vi "GFITS_Main.vi"() -> ()   [LabVIEW 2016]
doc: "Main VI for the TCS P60 interface"
uses:
  Common/public/vis/CMN_FVAR_action.ctl
  DBSHAND/private/vis/DatabaseHand_Element_Set(string).vi
  private/vis/GFITS_Gbls.vi
  DBSHAND/private/vis/DatabaseHand_Element_Get(string).vi
  DBSHAND/private/vis/DatabaseHand_Element_Get(bool).vi
  DBSHAND/private/vis/DatabaseHand_Element_Get(I32).vi
  DBSHAND/private/vis/DatabaseHand_Element_Set(I32).vi
  DBSHAND/private/vis/DatabaseHand_Element_Set(bool).vi
  DBSHAND/private/vis/DatabaseHand_Element_Get(path).vi
panel:
  in  "ignorename":string
  in  "testbname":string="test"
  in  "testdir":path=path "/tmp"
  out "tmpname":bool
  in  "postimg":string="none"
  in  "lognetfile":path
  in  "lognet":bool
  in  "defexts":bool=TRUE
  in  "imlog":bool
  in  "maxlistsize":i32=200
  in  "geomhdrmode":string="dynamic"
  in  "hdrmode":string="dynamic"
  in  "hdrprealloc":string="auto"
  in  "imnumformat":string="%04d"
  in  "waitstats":u32
  in  "preimg":string="none"
  in  "logfilepp":path
  in  "logpp":bool
  in  "postproc":string
  out "multiple extensions":bool
  out "after expid":string
  in  "filemsg":string
  in  "headers":bool=TRUE
  out "expID":string
  in  "asyncs":bool
  in  "imlogpath":path
  in  "cmdport2":u16=4062
  out "mImpath":string
  in  "nodeID":string
  in  "netenable":bool
  in  "cmdport":u16
  in  "saveconfig":bool
  out "image name out":string
  out "imretries":i32=20
  in  "log":bool
  in  "logfile":path
  in  "def_head_tim":string="after"
  out "amplifiers":u64
  in  "commands2exec":string
  in  "hdrfile":path
  out "ReadMode":string
  out "number of keywords":i32[](array[numeric])
  out "file reference":u64
  out "image size":u32
  in  "image data":T1
  in  "cmd struct":T2
  out "error out":errorcluster
  in  "Initialization Variables":string[][](table)=[["HDRFILE", "path", "GFITS_Main.vi", "hdrfile", "", "PATH"], ["HDRFILE", "prealloc", "GFITS_Main.vi", "hdrprealloc", "", "STR"], ["HDRFILE", "geommode", "GFITS_Main.vi", "geomhdrmode", "", "STR"], ["HDRFILE", "defmultext", "GFITS_Main.vi", "defexts", "", "BOOL"], ["HDRFILE", "mode", "GFITS_Main.vi", "hdrmode", "", "STR"], ["MISC", "commands", "GFITS_Main.vi", "commands2exec", "none", "STR"], ["MISC", "headtiming", "GFITS_Main.vi", "def_head_tim", "after", "STR"], ["MISC", "autosavecfg", "GFITS_Main.vi", "saveconfig", "", "BOOL"], ["MISC", "asyncmsg", "GFITS_Main.vi", "asyncs", "", "BOOL"], ["MISC", "filemsg", "GFITS_Main.vi", "filemsg", "", "STR"], ["MISC", "imnumformat", "GFITS_Main.vi", "imnumformat", "", "STR"], ["MISC", "testdir", "GFITS_Main.vi", "testdir", "", "PATH"], ["MISC", "testbname", "GFITS_Main.vi", "testbname", "", "STR"], ["MISC", "ignorename", "GFITS_Main.vi", "ignorename", "", "STR"], ["LOG", "file", "GFITS_Main.vi", "logfile", "none", "PATH"], ["LOG", "log", "GFITS_Main.vi", "log", "FALSE", "BOOL"], ["LOG", "imlogfile", "GFITS_Main.vi", "imlogpath", "", "PATH"], ["LOG", "imlog", "GFITS_Main.vi", "imlog", "", "BOOL"], ["LOG", "maxlistsize(kb)", "GFITS_Main.vi", "maxlistsize", "", "I32"], ["NetComms", "port", "GFITS_Main.vi", "cmdport", "", "U16"], ["NetComms", "port2", "GFITS_Main.vi", "cmdport2", "", "U16"], ["NetComms", "enable", "GFITS_Main.vi", "netenable", "", "BOOL"], ["NetComms", "log", "GFITS_Main.vi", "lognet", "", "BOOL"], ["NetComms", "logfile", "GFITS_Main.vi", "lognetfile", "", "PATH"], ["PostProc", "cmd", "GFITS_Main.vi", "postproc", "", "STR"], ["PostProc", "log", "GFITS_Main.vi", "logpp", "", "BOOL"], ["PostProc", "file", "GFITS_Main.vi", "logfilepp", "", "PATH"], ["PostImg", "cmd", "GFITS_Main.vi", "postimg", "", "STR"], ["PreImg", "cmd", "GFITS_Main.vi", "preimg", "", "STR"]]
  in  "error in":errorcluster
  out "ConfigFile":path=path "/home/ArcVIEW/Modules/TCSP60/config/TCSP60_Default.cfg"
  in  "ModuleName":string="GFITS"
  out "Command":string
  out "stopped":bool=TRUE
  out "Reply to":string
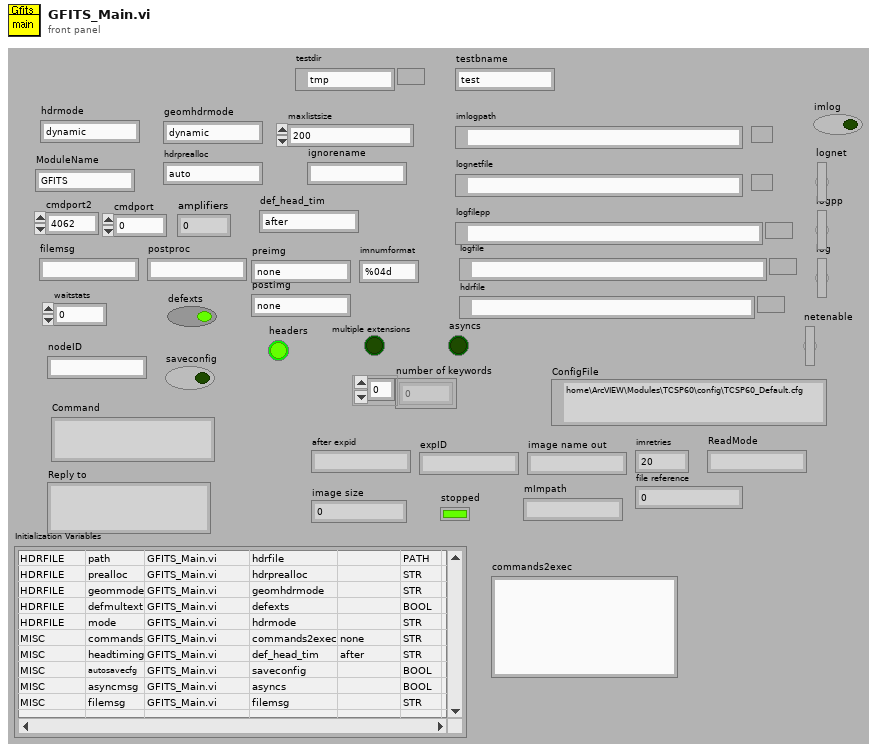
[diagram p1: front panel]
types:
  T1 = cluster{"location":u64, "eleRead":u32[], "data":u16[]}
  T2 = cluster{"command":string, "data":string, "responseQ":string, "nodeID":string}
  T3 = cluster{"name":string, "Path":path, "bitpix":i8, "naxis":u8, "naxes":u32[], "datatype":u16, "multiple extensions":bool, "hdutype":u16, "writeToDisk":bool, "num_of_ext":u8, "file ref":i32, "createnewimage":bool}
  T4 = typedef "CMN_FVAR_action.ctl" = enum16{"read", "write"}
  T5 = typedef "DatabaseHand_RefNum.ctl" = refnum<vi>
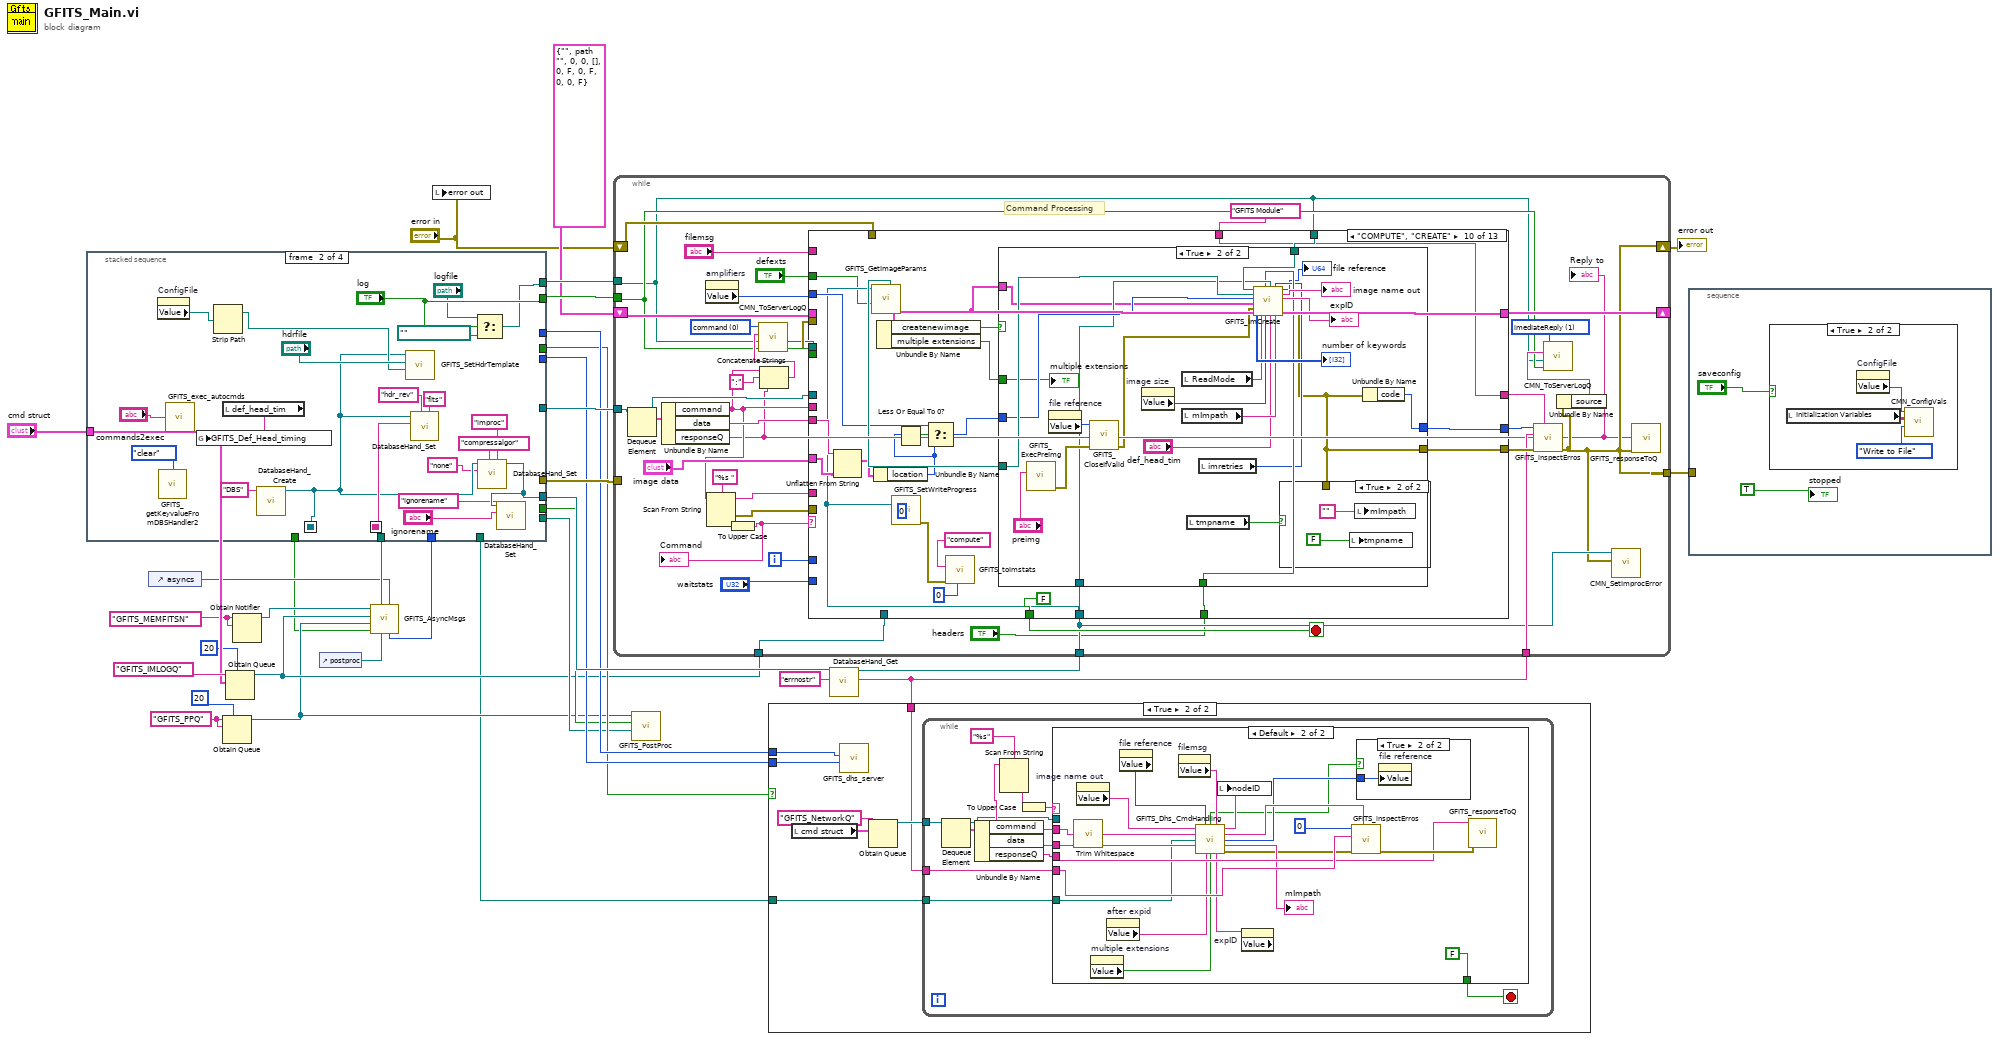
[diagram p0: block diagram]
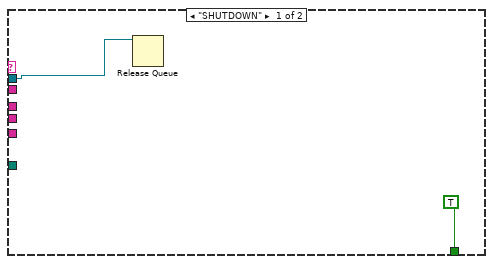
[diagram p3: hidden frame]
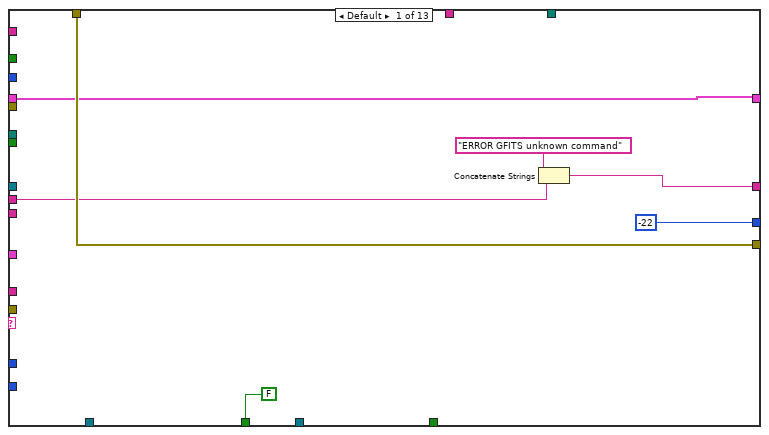
[diagram p6: hidden frame]
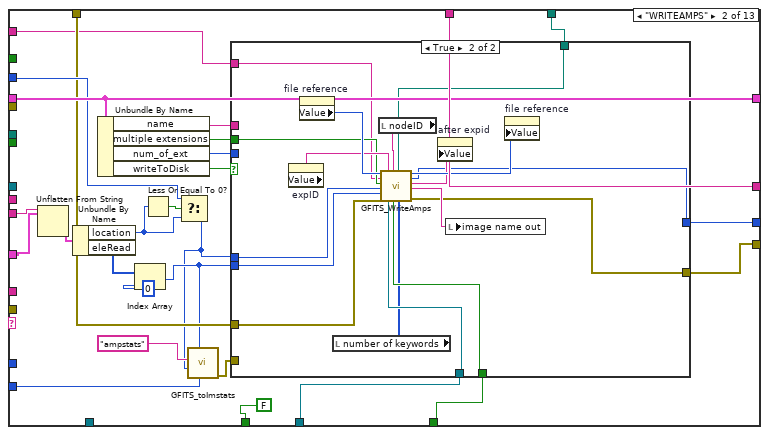
[diagram p7: hidden frame]
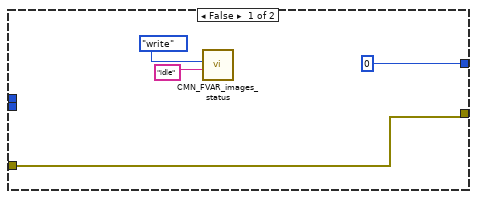
[diagram p8: hidden frame]
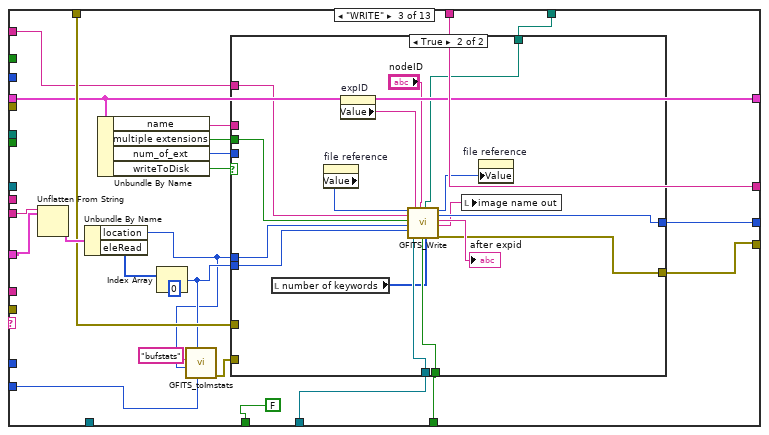
[diagram p9: hidden frame]
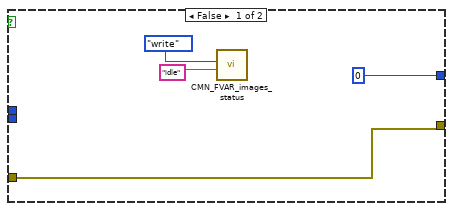
[diagram p10: hidden frame]
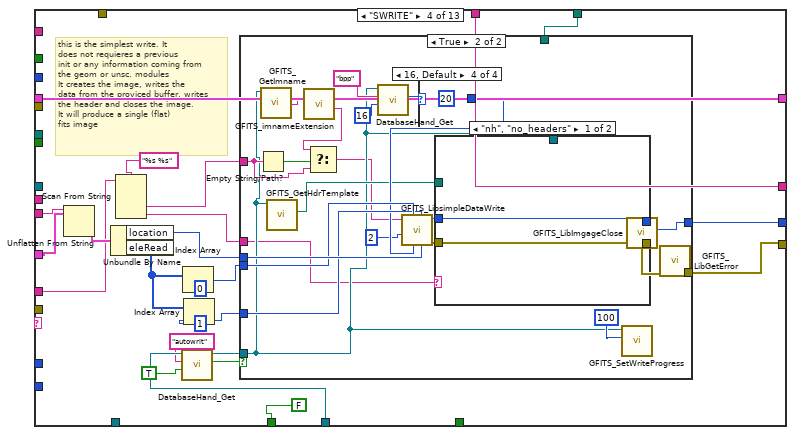
[diagram p11: hidden frame]
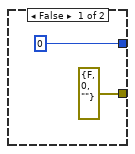
[diagram p12: hidden frame]
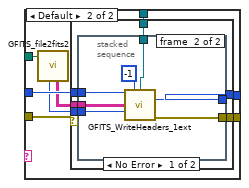
[diagram p13: hidden frame]
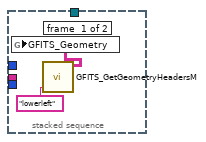
[diagram p14: hidden frame]
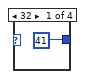
[diagram p16: hidden frame]
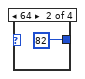
[diagram p17: hidden frame]
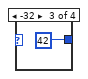
[diagram p18: hidden frame]
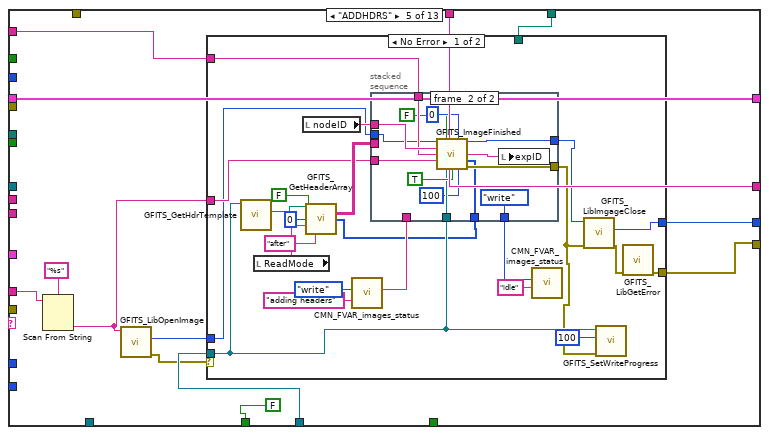
[diagram p19: hidden frame]
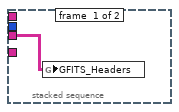
[diagram p20: hidden frame]
diagram:
  w14 = "GFITS_PPQ" ("name (unnamed)")
  w16 = "GFITS_MEMFITSN" ("name (unnamed)")
  n1 = stacked-sequence {
    seq-local: [w39 _ _ _] -> [_ w57 _ _]
    seq-local: [_ w50 _ _] -> [_ _ w69 _]
    tunnel: [w36 _ _ _] -> w32
    tunnel: [_ w48 _ _] -> w31
    tunnel: [_ "log" _ _] -> w30
    tunnel: [_ w60 _ _] -> w29
    tunnel: [w37 _ _ _] -> w28
    tunnel: [_ _ "cmdport" _] -> w21
    tunnel: [_ _ "netenable" _] -> w20
    tunnel: [_ _ "cmdport2" _] -> w22
    tunnel: [_ _ "imlogpath" _] -> w8
    tunnel: "cmd struct" -> [w35 _ _ _]
    tunnel: [_ _ "logpp" _] -> w13
    tunnel: [_ _ "logfilepp" _] -> w12
    tunnel: [_ _ w79 _] -> w3
    tunnel: [_ _ "imlog" _] -> w2
    tunnel: [_ _ _ "lognetfile"] -> w1
    frame #0 {
      # "Initialization"
      n2 = call "CMN_FVAR_images_status.vi"("value in"="idle", "action"=CMN_FVAR_action."write") -> ()  [unwired: 9 out]
      n3 = Current VI's Path() -> (path=w41:path)
      n4 = call "CMN_testpath.vi"("ModuleName"="ModuleName", "caller Path"=w41) -> ("ConfigFile"=w43:path)  [unwired: 1 in, 8 out]
      "ConfigFile" <- w43
      n5 = local write "stopped"(FALSE ("stopped")) -> ()
      n6 = call "CMN_modinfo.vi"("full"=FALSE, "caller path"=w41) -> ("INFO"=w39:string)  [unwired: 1 in, 8 out]
      n7 = Obtain Queue(name (unnamed)="GFITS_INTERNALQ", element data type=w35) -> (queue out=w37:refnum<queue>, error out=w36:errorcluster)  [unwired: 3 in, 1 out]
      n8 = call "CMN_ConfigVals.vi"("ConfigVariables"="Initialization Variables", "configuration file path"=w43) -> ()  [unwired: 2 in, 8 out]
    }
    frame #1 {
      n9 = property on="ConfigFile" class="Path"() -> ("Value"=w54:path)  [unwired: 2 in, 2 out]
      n10 = call "GFITS_getKeyvalueFromDBSHandler2.vi"("action"=enum16{"get", "clear"}."clear") -> ()  [unwired: 8 in, 7 out]
      n11 = call "GFITS_exec_autocmds.vi"("commands2exec"="commands2exec") -> ()
      n12 = Strip Path(path=w54) -> (stripped path=w53:path)  [unwired: 1 out]
      n13 = local read "def_head_tim"() -> (w56:string)
      n14 = global write "GFITS_Gbls.vi" "GFITS_Def_Head_timing"(w56) -> ()
      n15 = call "DatabaseHand_Create.vi"("Name"="DBS") -> ("Database RefNum out"=w50:T5)  [unwired: 1 in, 9 out]
      n16 = call "GFITS_SetHdrTemplate.vi"("ref path"=w53, "path"="hdrfile", "Database RefNum"=w50) -> ()  [unwired: 9 out]
      n17 = call-poly "DatabaseHand_Set.vi"("group"="fits", "name"="hdr_rev", "value"=w57, "Database RefNum in"=w50) -> ()  [unwired: 4 in, 4 out]
      n18 = Select(t="logfile", s="log", f=path "") -> (s? t:f=w60:path)
      n19 = call-poly "DatabaseHand_Set.vi"("group"="improc", "name"="compressalgor", "value"="none", "Database RefNum in"=w50) -> ("Database RefNum out"=w48:T5)  [unwired: 4 in, 3 out]
      n20 = call-poly "DatabaseHand_Set.vi"("name"="ignorename", "value"="ignorename", "Database RefNum in"=w48) -> ()  [unwired: 5 in, 4 out]
    }
    frame #2 {
      n21 = property on="preimg" class="Str"() -> ("Value"=w73:string)  [unwired: 2 in, 2 out]
      n22 = call "GFITS_ParsePostProc.vi"("postproc in"=w73) -> ("postproc out"=w72:string)  [unwired: 10 out]
      n23 = call "GFITS_ParsePostProc.vi"("postproc in"="postproc") -> ("postproc out"=w75:string)  [unwired: 10 out]
      n24 = call "GFITS_ParsePostProc.vi"("postproc in"="postimg") -> ("postproc out"=w71:string)  [unwired: 10 out]
      n25 = case shown="False" "lognet" {
        frame False {
          n26 = property on="lognetfile" class="Path"("Value"=path "") -> ()  [unwired: 2 in, 2 out]
        }
        frame True {
        }
      }
      n27 = property on="postproc" class="Str"("Value"=w75) -> ()  [unwired: 2 in, 2 out]
      n28 = property on="preimg" class="Str"("Value"=w72) -> ()  [unwired: 2 in, 2 out]
      n29 = call "GFITS_VAR_postImgScript.vi"("script name in"=w71, "action"=enum16{"read", "write"}."write") -> ()  [unwired: 14 out]
      n30 = call "GFITS_SetImNumFormat.vi"("imnumformat"="imnumformat", "Database RefNum out"=w69) -> ()  [unwired: 1 in, 9 out]
      n31 = call "GFITS_LibInitExtensions.vi"() -> ()  [unwired: 1 in, 11 out]
      n32 = Multiply(x="maxlistsize", y=1024) -> (x*y=w79:i32)
      n33 = call "GFITS_SetTestVars.vi"("testbname"="testbname", "testdir"="testdir", "Database RefNum in"=w69) -> ()  [unwired: 9 out]
    }
    frame #3 {
      n34 = call <vilib>:"Trim Whitespace.vi"("string"="geomhdrmode") -> ("trimmed string"=w92:string)  [unwired: 1 in]
      n35 = call <vilib>:"Trim Whitespace.vi"("string"="hdrmode") -> ("trimmed string"=w99:string)  [unwired: 1 in]
      n36 = call <vilib>:"Trim Whitespace.vi"("string"="hdrprealloc") -> ("trimmed string"=w101:string)  [unwired: 1 in]
      n37 = To Lower Case(string=w92) -> (all lower case string=w91:string)
      n38 = To Lower Case(string=w99) -> (all lower case string=w100:string)
      n39 = To Lower Case(string=w101) -> (all lower case string=w105:string)
      n40 = case shown="\"\", \"auto\", \"dynamic\", Default" w91 {
        tunnel: w92 -> [_ _]
        tunnel: [TRUE ("nkeys in") FALSE ("nkeys in")] -> w95
        frame "static" {
        }
        frame "", "auto", "dynamic", Default {
        }
      }
      n41 = case shown="\"\", \"auto\", \"dynamic\"" w105 {
        tunnel: [w111 -1 ("nkeys in")] -> w103
        tunnel: w101 -> [w114 _]
        frame Default {
          n42 = Scan From String(format string="%d", input string=w114) -> (error out=w113:errorcluster, output 1=w112:i32)  [unwired: 2 in, 3 out]
          n43 = Select(t=-1, s=w113, f=w112) -> (s? t:f=w111:i32)
        }
        frame "", "auto", "dynamic" {
        }
      }
      n44 = case shown="\"\", \"auto\", \"dynamic\", Default" w100 {
        tunnel: w99 -> [_ _]
        tunnel: [TRUE ("nkeys in") FALSE ("nkeys in")] -> w96
        frame "static" {
        }
        frame "", "auto", "dynamic", Default {
        }
      }
      n45 = call "GFITS_VAR_fstaticGeomHdrs.vi"("static in"=w95, "action"=enum16{"read", "write"}."write") -> ()  [unwired: 14 out]
      n46 = call "GFITS_VAR_staticHdrs.vi"("static in"=w96, "action"=enum16{"read", "write"}."write") -> ()  [unwired: 14 out]
      n47 = call "GFITS_VAR_preallocHdrs.vi"("nkeys in"=w103, "action"=enum16{"read", "write"}."write") -> ()  [unwired: 14 out]
    }
  }
  n48 = control-ref of="asyncs"() -> (w7:refnum<vi>)
  n49 = Obtain Queue(max queue size (-1, unlimited)=20, name (unnamed)=w14, element data type=w14) -> (queue out=w9:refnum<queue>)  [unwired: 2 in, 2 out]
  n50 = Obtain Queue(max queue size (-1, unlimited)=20, name (unnamed)="GFITS_IMLOGQ", element data type="cmd struct") -> (queue out=w10:refnum<queue>)  [unwired: 2 in, 2 out]
  n51 = Obtain Notifier(name (unnamed)=w16, notification data type=w16) -> (notifier out=w11:refnum<notifier>)  [unwired: 2 in, 2 out]
  n52 = control-ref of="postproc"() -> (w6:refnum<vi>)
  n53 = call "GFITS_AsyncMsgs.vi"("max imlist size"=w3, "asyncs"=w7, "postproc"=w6, "imlogs"=w8, "imlog"=w2, "PPQ"=w9, "imlogq"=w10, "notifier in"=w11) -> ()  [unwired: 4 out]
  n54 = local write "error out"("error in") -> ()
  n55 = call "GFITS_PostProc.vi"("logpath"=w12, "log"=w13, "queue in"=w9) -> ()  [unwired: 9 out]
  n56 = call-poly "DatabaseHand_Get.vi"("name"="errnostr", "Database RefNum in"=w31) -> ("value"=w19:string, "Database RefNum out"=w24:T5)  [unwired: 3 in, 5 out]
  n57 = while {
    tunnel: w32 -> [_]
    shift-right: [w124] -> w26
    shift-left: "error in" -> [w147]
    shift-right: [w139] -> _
    shift-left: T3 {"name"="", "Path"=path "", "bitpix"=0, "naxis"=0, "naxes"=[], "datatype"=0, "multiple extensions"=FALSE, "hdutype"=0, "writeToDisk"=FALSE, "num_of_ext"=0, "file ref"=0, "createnewimage"=FALSE} ("imageStruct") -> [w141]
    tunnel: [w124] -> w25
    tunnel: w24 -> [w136]
    tunnel: w19 -> [w137]
    tunnel: w29 -> [w128]
    tunnel: w30 -> [w130]
    tunnel: w28 -> [w127]
    tunnel: w10 -> [w121]
    i -> [w153]
    stop <- w154 stop-if-true
    w134 = u16 1 items=["command", "imediateReply", "Callback Reply", "Information"] ("type")
    w135 = u16 0 items=["command", "imediateReply", "Callback Reply", "Information"] ("type")
    # "Command Processing"
    n58 = Dequeue Element(queue=w127) -> (queue out=w125:refnum<queue>, element=w126:T2)  [unwired: 1 in, 3 out]
    n59 = Unbundle By Name(w126) -> ("command"=w123:string, "data"=w145:string, "responseQ"=w122:string)
    "Reply to" <- w122
    n60 = property on="amplifiers" class="DigNum (strict)"() -> ("Value"=w138:u64)  [unwired: 2 in, 2 out]
    n61 = Scan From String(format string="%s ", input string=w123) -> (remaining string=w149:string, error out=w151:errorcluster, output 1=w150:string)  [unwired: 2 in, 2 out]
    n62 = To Upper Case(1:w150) -> (0:w148:string)
    "Command" <- w148
    n63 = Concatenate Strings(w123, ":" ("string"), w122) -> (w132:string)
    n64 = call "CMN_ToServerLogQ.vi"("Log"=w130, "file"=w128, "string"=w132, "type"=w135) -> ("error out"=w129:errorcluster)  [unwired: 2 in, 4 out]
    n65 = case shown="\"COMPUTE\", \"CREATE\"" w148 {
      selector: w148 -> [_ _ _ _ _ _ w423 _ _ _ _ _ _]
      tunnel: [FALSE FALSE FALSE FALSE FALSE FALSE TRUE FALSE FALSE FALSE FALSE FALSE FALSE] -> w154
      tunnel: w151 -> [_ _ _ _ _ _ _ _ _ _ _ _ _]
      tunnel: w153 -> [_ _ _ _ _ _ _ _ _ _ _ _ _]
      tunnel: w149 -> [_ _ _ w257 w339 _ _ _ w453 _ _ _ w1126]
      tunnel: w147 -> [w159 w170 w227 _ _ _ w434 w447 w463 _ _ _ w1124]
      tunnel: [w159 w180 w224 w270 w344 w398 w433 w447 w464 w1049 errorcluster {"status"=FALSE, "code"=0, "source"=""} ("error out") errorcluster {"status"=FALSE, "code"=0, "source"=""} ("error out") w1122] -> w146
      tunnel: w145 -> [_ w188 w233 w277 _ w419 _ _ w455 w1045 _ _ _]
      tunnel: [-22 w182 w226 w272 w346 w416 w432 0 w451 w1048 0 ("return value") 0 ("return value") w1123] -> w144
      tunnel: w123 -> [w157 _ _ _ _ _ _ _ _ _ _ _ _]
      tunnel: "GFITS Module" ("message") -> [_ w181 w225 w271 w345 w420 w436 w442 _ w1029 _ _ _]
      tunnel: [w156 w181 w225 w271 w345 w420 w436 w440 w457 w1029 "aborting write" ("message") "done" ("message") w1121] -> w142
      tunnel: [w155 w179 w223 w269 w343 w403 w435 w439 w465 w1030 w1098 w1109 w1120] -> w139
      tunnel: w141 -> [w155 w179 w223 w269 w343 _ w435 w439 w466 _ w1098 w1109 w1120]
      tunnel: "image data" -> [_ w186 w231 w275 _ w418 _ _ _ w1046 _ _ _]
      tunnel: w138 -> [_ w173 _ _ _ _ _ _ _ w1041 _ _ _]
      tunnel: w136 -> [_ w172 w218 w262 w341 w404 w431 _ w462 w1038 _ w1104 _]
      tunnel: w128 -> [_ _ _ _ _ _ _ _ w460 _ _ _ _]
      tunnel: w130 -> [_ _ _ _ _ _ _ _ w459 _ _ _ _]
      tunnel: w129 -> [_ _ _ _ _ _ _ _ w458 _ _ _ _]
      tunnel: w128 -> [_ w171 w217 w268 w342 _ _ _ _ w1037 _ _ _]
      tunnel: w125 -> [_ _ _ _ _ _ w426 _ _ _ _ _ _]
      tunnel: w121 -> [_ _ _ _ _ _ w425 _ _ _ _ _ _]
      tunnel: "headers" -> [_ w162 w216 _ _ _ _ _ _ w1034 _ _ _]
      tunnel: "filemsg" -> [_ w169 w215 _ w340 _ _ _ w452 _ _ w1105 _]
      tunnel: "waitstats" -> [_ w165 w213 _ _ _ _ _ _ _ _ _ _]
      tunnel: "defexts" -> [_ _ _ _ _ w390 _ _ w450 w1028 _ _ _]
      frame Default {
        n66 = Concatenate Strings("ERROR GFITS unknown command", w157) -> (w156:string)
      }
      frame "WRITEAMPS" {
        n67 = Unflatten From String(type=w186, binary string=w188) -> (value=w185:T1)  [unwired: 1 in, 4 out]
        n68 = Unbundle By Name(w185) -> ("location"=w167:u64, "eleRead"=w184:u32[])
        n69 = Unbundle By Name(w179) -> ("name"=w178:string, "multiple extensions"=w176:bool, "num_of_ext"=w177:u8, "writeToDisk"=w175:bool)
        n70 = Index Array(array=w184, index=0) -> (element=w164:u32)
        n71 = Less Or Equal To 0?(x=w167) -> (x <= 0?=w174:bool)
        n72 = Select(t=w173, s=w174, f=w167) -> (s? t:f=w163:u64)
        n73 = call "GFITS_toImstats.vi"("wait"=w165, "nelems"=w164, "ptr"=w163, "cmd"="ampstats") -> ("error out"=w166:errorcluster)  [unwired: 1 in, 6 out]
        n74 = case shown="True" w175 {
          tunnel: w163 -> [_ w205]
          tunnel: w164 -> [_ w204]
          tunnel: w170 -> [w192 w203]
          tunnel: [0 ("return value") w194] -> w182
          tunnel: [w192 w193] -> w180
          tunnel: w178 -> [_ _]
          tunnel: w177 -> [_ _]
          tunnel: w176 -> [_ w206]
          tunnel: w172 -> [_ w200]
          tunnel: w171 -> [_ w201]
          tunnel: w162 -> [_ w199]
          tunnel: w169 -> [_ w202]
          tunnel: w166 -> [_ _]
          frame False {
            n75 = call "CMN_FVAR_images_status.vi"("value in"="idle", "action"=CMN_FVAR_action."write") -> ()  [unwired: 9 out]
          }
          frame True {
            n76 = property on="expID" class="Str"() -> ("Value"=w208:string)  [unwired: 2 in, 2 out]
            n77 = property on="file reference" class="DigNum (strict)"() -> ("Value"=w209:u64)  [unwired: 2 in, 2 out]
            n78 = local read "number of keywords"() -> (w198:i32[])
            n79 = local read "nodeID"() -> (w207:string)
            n80 = call "GFITS_WriteAmps.vi"("fd"=w209, "filemsg"=w202, "multimple extensions"=w206, "amplifiers"=w205, "eleRead"=w204, "error in"=w203, "expID"=w208, "Database RefNum in"=w200, "nodeID"=w207, "headers"=w199, "logfile"=w201, "number of keywords"=w198) -> ("file reference out"=w197:u64, "return value"=w194:i32, "after expID"=w195:string, "image name out"=w196:string, "error out"=w193:errorcluster)  [unwired: 3 out]
            n81 = property on="after expid" class="Str"("Value"=w195) -> ()  [unwired: 2 in, 2 out]
            n82 = local write "image name out"(w196) -> ()
            n83 = property on="file reference" class="DigNum (strict)"("Value"=w197) -> ()  [unwired: 2 in, 2 out]
          }
        }
      }
      frame "WRITE" {
        n84 = Unflatten From String(type=w231, binary string=w233) -> (value=w230:T1)  [unwired: 1 in, 4 out]
        n85 = Unbundle By Name(w230) -> ("location"=w210:u64, "eleRead"=w229:u32[])
        n86 = Unbundle By Name(w223) -> ("name"=w222:string, "multiple extensions"=w220:bool, "num_of_ext"=w221:u8, "writeToDisk"=w219:bool)
        n87 = Index Array(array=w229, index=0) -> (element=w211:u32)
        n88 = call "GFITS_toImstats.vi"("wait"=w213, "nelems"=w211, "ptr"=w210, "cmd"="bufstats") -> ("error out"=w212:errorcluster)  [unwired: 1 in, 6 out]
        n89 = case shown="True" w219 {
          tunnel: w210 -> [_ w250]
          tunnel: w211 -> [_ w249]
          tunnel: w227 -> [w237 _]
          tunnel: [0 ("return value") w241] -> w226
          tunnel: [w237 w240] -> w224
          tunnel: w222 -> [_ _]
          tunnel: w221 -> [_ _]
          tunnel: w220 -> [_ w251]
          tunnel: w218 -> [_ w247]
          tunnel: w217 -> [_ w242]
          tunnel: w216 -> [_ w246]
          tunnel: w215 -> [_ w252]
          tunnel: w212 -> [_ _]
          frame False {
            n90 = call "CMN_FVAR_images_status.vi"("value in"="idle", "action"=CMN_FVAR_action."write") -> ()  [unwired: 9 out]
          }
          frame True {
            n91 = local read "number of keywords"() -> (w245:i32[])
            n92 = property on="file reference" class="DigNum (strict)"() -> ("Value"=w253:u64)  [unwired: 2 in, 2 out]
            n93 = property on="expID" class="Str"() -> ("Value"=w244:string)  [unwired: 2 in, 2 out]
            n94 = call "GFITS_Write.vi"("fd"=w253, "filemsg"=w252, "multimple extensions"=w251, "buffer"=w250, "eleRead"=w249, "expID"=w244, "Database RefNum in"=w247, "nodeID"="nodeID", "headers"=w246, "logfile"=w242, "number of keywords"=w245) -> ("file reference out"=w239:u64, "return value"=w241:i32, "after expID"=→"after expid":string, "image name out"=w238:string, "error out"=w240:errorcluster)  [unwired: 1 in, 3 out]
            n95 = local write "image name out"(w238) -> ()
            n96 = property on="file reference" class="DigNum (strict)"("Value"=w239) -> ()  [unwired: 2 in, 2 out]
          }
        }
      }
      frame "SWRITE" {
        # "this is the simplest write. It\ndoes not requieres a previous\ninit or any information coming from\nthe geom or unsc. modules\nIt creates the image, writes the\ndata from the proviced buffer, writes\nthe header and closes the image.\nIt will produce a single (flat)\nfits image"
        n97 = Unflatten From String(type=w275, binary string=w277) -> (value=w274:T1)  [unwired: 1 in, 4 out]
        n98 = Unbundle By Name(w274) -> ("location"=w266:u64, "eleRead"=w264:u32[])
        n99 = Scan From String(format string="%s %s", input string=w257) -> (output 1=w255:string, output 2=w254:string)  [unwired: 2 in, 5 out]
        n100 = call-poly "DatabaseHand_Get.vi"("default value"=TRUE, "name"="autowrit", "Database RefNum in"=w262) -> ("value"=w259:bool, "Database RefNum out"=w258:T5)  [unwired: 2 in, 5 out]
        n101 = Index Array(array=w264, index=0) -> (element=w267:u32)
        n102 = Index Array(array=w264, index=1) -> (element=w263:u32)
        n103 = case shown="True" w259 {
          tunnel: w266 -> [_ w301]
          tunnel: w267 -> [_ w300]
          tunnel: [0 ("return value") w289] -> w272
          tunnel: [errorcluster {"status"=FALSE, "code"=0, "source"=""} ("error out") w303] -> w270
          tunnel: w268 -> [_ _]
          tunnel: w263 -> [_ w299]
          tunnel: w258 -> [_ w284]
          tunnel: w255 -> [_ w285]
          tunnel: w254 -> [_ w280]
          frame False {
          }
          frame True {
            n104 = Empty String/Path?(string/path=w285) -> (empty?=w286:bool)
            n105 = call "GFITS_GetImname.vi"("Database RefNum"=w284) -> ("name"=w287:string)  [unwired: 10 out]
            n106 = call "GFITS_GetHdrTemplate.vi"("Database RefNum"=w284) -> ("path"=w294:path)  [unwired: 10 out]
            n107 = call "GFITS_imnameExtension.vi"("imname in"=w287) -> ("rootname (no extension)"=w283:string)  [unwired: 9 out]
            n108 = Select(t=w283, s=w286, f=w285) -> (s? t:f=w282:string)
            n109 = call-poly "DatabaseHand_Get.vi"("default value"=16, "name"="bpp", "Database RefNum in"=w284) -> ("value"=w296:i32)  [unwired: 2 in, 6 out]
            n110 = case shown="16, Default" w296 {
              tunnel: [41 82 42 20] -> w295
              frame 32 {
              }
              frame 64 {
              }
              frame -32 {
              }
              frame 16, Default {
              }
            }
            n111 = call "GFITS_LibsimpleDataWrite.vi"("bufptr"=w301, "nrows"=w299, "dtype"=w295, "ncols"=w300, "ntries"=2, "name"=w282) -> ("error out"=w288:errorcluster, "ref out"=w293:u64)  [unwired: 1 in, 3 out]
            n112 = case shown="\"nh\", \"no_headers\"" w280 {
              tunnel: w294 -> [_ w313]
              tunnel: w293 -> [w305 w312]
              tunnel: [w305 w309] -> w292
              tunnel: [w304 w308] -> w291
              tunnel: w288 -> [w304 w307]
              tunnel: w284 -> [_ w306]
              frame "nh", "no_headers" {
              }
              frame Default {
                n113 = call "GFITS_file2fits2.vi"("file"=w313) -> ("all keys"=w311:string[][], "number of total keywords"=w310:i32)  [unwired: 1 in, 8 out]
                n114 = case shown="No Error" w307 {
                  selector: w307 -> [_ w329]
                  tunnel: w312 -> [w319 w330]
                  tunnel: w311 -> [w318 _]
                  tunnel: w306 -> [w317 _]
                  tunnel: w310 -> [w316 _]
                  tunnel: [w315 w330] -> w309
                  tunnel: [w314 w329] -> w308
                  frame No Error {
                    n115 = stacked-sequence {
                      tunnel: w319 -> [_ w328]
                      tunnel: w318 -> [_ w326]
                      tunnel: w317 -> [_ w325]
                      tunnel: w316 -> [_ w324]
                      tunnel: [_ w323] -> w315
                      tunnel: [_ w322] -> w314
                      frame #0 {
                        n116 = call "GFITS_GetGeometryHeadersM.vi"("readmode"="lowerleft") -> ("Keywords out"=w321:string[][][])  [unwired: 10 out]
                        n117 = global write "GFITS_Gbls.vi" "GFITS_Geometry"(w321) -> ()
                      }
                      frame #1 {
                        n118 = call "GFITS_WriteHeaders_1ext.vi"("ref"=w328, "extension"=-1, "Database RefNum in"=w325, "Keywords"=w326, "numer of keywords"=w324) -> ("ref out"=w323:u64, "error out"=w322:errorcluster)  [unwired: 2 in, 7 out]
                      }
                    }
                  }
                  frame Error {
                  }
                }
              }
            }
            n119 = call "GFITS_SetWriteProgress.vi"("progress"=100, "Database RefNum"=w284) -> ()  [unwired: 1 in, 9 out]
            n120 = call "GFITS_LibImgageClose.vi"("error in (no error)"=w291, "fd"=w292) -> ("error out"=w290:errorcluster, "return value"=w289:i32)  [unwired: 1 in, 7 out]
            n121 = call "GFITS_LibGetError.vi"("error in (no error)"=w290) -> ("error out"=w303:errorcluster)  [unwired: 10 out]
          }
        }
      }
      frame "ADDHDRS" {
        n122 = Scan From String(format string="%s", input string=w339) -> (output 1=w337:string)  [unwired: 2 in, 4 out]
        n123 = call "GFITS_LibOpenImage.vi"("imname"=w337) -> ("error out"=w335:errorcluster, "return value"=w336:u64)  [unwired: 1 in, 8 out]
        n124 = case shown="No Error" w335 {
          tunnel: [w368 0 ("return value")] -> w346
          tunnel: [w370 errorcluster {"status"=FALSE, "code"=0, "source"=""} ("error out")] -> w344
          tunnel: w342 -> [_ _]
          tunnel: w341 -> [w359 _]
          tunnel: w340 -> [w360 _]
          tunnel: w337 -> [w352 _]
          tunnel: w336 -> [w351 _]
          frame No Error {
            n125 = call "GFITS_GetHdrTemplate.vi"("Database RefNum"=w359) -> ("path"=w367:path)  [unwired: 10 out]
            n126 = local read "ReadMode"() -> (w366:string)
            n127 = local read "nodeID"() -> (w361:string)
            n128 = call "GFITS_GetHeaderArray.vi"("file"=w367, "mext"=FALSE, "number of Extensions"=u16 0, "readmode"=w366, "def_timing"="after") -> ("After keys"=w362:string[][][], "number of after keywords"=w348:i32[])  [unwired: 2 in, 7 out]
            n129 = call "CMN_FVAR_images_status.vi"("value in"="adding headers", "action"=CMN_FVAR_action."write") -> ("value out"=w356:string)  [unwired: 8 out]
            n130 = stacked-sequence {
              tunnel: w362 -> [w371 _]
              tunnel: w361 -> [_ w383]
              tunnel: w360 -> [_ w382]
              tunnel: w359 -> [_ w379]
              tunnel: [_ w378] -> w355
              tunnel: w356 -> [_ _]
              tunnel: [_ CMN_FVAR_action."write" ("action")] -> w354
              tunnel: w352 -> [_ w376]
              tunnel: w351 -> [_ w375]
              tunnel: [_ w374] -> w350
              tunnel: w348 -> [_ w372]
              frame #0 {
                n131 = global write "GFITS_Gbls.vi" "GFITS_Headers"(w371) -> ()
              }
              frame #1 {
                n132 = call "GFITS_ImageFinished.vi"("file reference"=w375, "multimple extensions"=FALSE, "num of extensions"=u16 0, "nodeID"=w383, "filemsg"=w382, "image name"=w376, "number of keywords"=w372, "Database RefNum in"=w379, "headers"=TRUE, "progress"=i16 100) -> ("file reference out"=w374:u64, "expID"=w384:string, "error out"=w378:errorcluster)  [unwired: 3 in]
                n133 = local write "expID"(w384) -> ()
              }
            }
            n134 = call "CMN_FVAR_images_status.vi"("value in"="idle", "action"=w354) -> ()  [unwired: 9 out]
            n135 = call "GFITS_LibImgageClose.vi"("error in (no error)"=w355, "fd"=w350) -> ("error out"=w369:errorcluster, "return value"=w368:i32)  [unwired: 1 in, 7 out]
            n136 = call "GFITS_SetWriteProgress.vi"("error in (no error)"=w355, "progress"=100, "Database RefNum"=w359) -> ()  [unwired: 9 out]
            n137 = call "GFITS_LibGetError.vi"("error in (no error)"=w369) -> ("error out"=w370:errorcluster)  [unwired: 10 out]
          }
          frame Error {
            n138 = call "CMN_FVAR_images_status.vi"("value in"="idle", "action"=CMN_FVAR_action."write") -> ()  [unwired: 9 out]
          }
        }
      }
      frame "INIT" {
        n139 = Unflatten From String(type=w418, binary string=w419) -> (value=w417:T1)  [unwired: 1 in, 4 out]
        n140 = call "GFITS_GetImageParams.vi"("defexts"=w390, "Database RefNum"=w404) -> ("imageStruct"=w403:T3, "CurrentReadMode"=w391:string, "header template"=w394:path)  [unwired: 7 out]
        "ReadMode" <- w391
        n141 = Unbundle By Name(w417) -> ("location"=w396:u64)
        "amplifiers" <- w396
        n142 = Unbundle By Name(w403) -> ("num_of_ext"=w395:u8, "multiple extensions"=w392:bool, "datatype"=w415:u16, "hdutype"=w414:u16, "naxes"=w412:u32[], "bitpix"=w402:i8)
        n143 = property on="def_head_tim" class="Str"() -> ("Value"=w393:string)  [unwired: 2 in, 2 out]
        n144 = Index Array(array=w412, index=0) -> (element=w410:u32)
        n145 = Index Array(array=w412, index=1) -> (element=w409:u32)
        n146 = Divide(x=w402, y=i8 8) -> (x/y=w400:dbl)
        n147 = call "GFITS_FillHdrGbl.vi"("mext"=w392, "ReadMode"=w391, "number of Extensions"=w395, "def_timing"=w393, "hdrfile"=w394) -> ()  [unwired: 7 out]
        n148 = call "GFITS_LibInit.vi"("totalrows"=w409, "namp"=w395, "totalcols"=w410, "amplifiers"=w396, "multiple extensions?"=w392, "hdutype"=w414, "datatype"=w415) -> ("error out"=w405:errorcluster, "return value"=w416:i32)  [unwired: 1 in, 2 out]
        n149 = To Unsigned Word Integer(number=w400) -> (unsigned 16bit integer=w407:u16)
        n150 = Compound Arithmetic op=MULTIPLY(w410, w409, w407) -> (w408:u32)
        n151 = call "GFITS_LibGetError.vi"("error in (no error)"=w405) -> ("error out"=w398:errorcluster)  [unwired: 10 out]
        n152 = To Unsigned Long Integer(number=w408) -> (unsigned 32bit integer=→"image size":u32)
        n153 = call "GFITS_toImstats.vi"("wait"=u32 0 ("ptr"), "error in (no error)"=w398, "ptr"=w396, "cmd"="INIT") -> ()  [unwired: 1 in, 7 out]
      }
      frame "SHUTDOWN" {
        w429 = "GFITS_COMS_SHUTDOWCmd_N" ("name (unnamed)")
        n154 = Release Queue(queue=w426) -> ()  [unwired: 1 in, 4 out]
        n155 = property on="cmd struct" class="Clust (strict)"() -> ("Value"=w424:T2)  [unwired: 2 in, 2 out]
        n156 = Bundle By Name(cluster=w424, "command"=w423) -> (w422:T2)
        n157 = Enqueue Element(queue=w425, element=w422) -> ()  [unwired: 1 in, 4 out]
        n158 = Obtain Notifier(name (unnamed)=w429, notification data type=w429) -> (notifier out=w428:refnum<notifier>)  [unwired: 2 in, 2 out]
        n159 = local write "stopped"(TRUE ("stopped")) -> ()
        n160 = Send Notification(notification="SERVER_SHUTDOWN", notifier=w428) -> ()  [unwired: 1 in, 2 out]
        n161 = call "GFITS_GetHdrTemplate.vi"("Database RefNum"=w431) -> ("path"=w430:path)  [unwired: 10 out]
        n162 = call "GFITS_LibClose.vi"("error in (no error)"=w434) -> ("error out"=w433:errorcluster, "return value"=w432:i32)  [unwired: 9 out]
        n163 = property on="hdrfile" class="Path"("Value"=w430) -> ()  [unwired: 2 in, 2 out]
      }
      frame "STATE" {
        n164 = Unbundle By Name(w447) -> ("source"=w445:string)
        n165 = Concatenate Strings("ERROR ", w445) -> (w444:string)
        n166 = Select(t=w444, s=w447, f="OK") -> (s? t:f=w441:string)
        n167 = Concatenate Strings(w442, w441) -> (w440:string)
      }
      frame "WRITEKEY" {
        w461 = u16 0 items=["command", "imediateReply", "Callback Reply", "Information"] ("type")
        n168 = call "CMN_ToServerLogQ.vi"("error in (no error)"=w458, "Log"=w459, "file"=w460, "string"=w455, "type"=w461) -> ()  [unwired: 1 in, 5 out]
        n169 = Scan From String(format string="%s" ("Format String"), input string=w455) -> (remaining string=w467:string, output 1=w468:string)  [unwired: 2 in, 3 out]
        n170 = case shown="\"bpp\"" w468 {
          tunnel: w467 -> [_ _ w498 w504 w513 w522 w524 w540 w552 w564 w567 w579 w591 w602 w615 w628 w640 w645 w661 w664 w683 w691 w706 _ _ _ _ _ _ _ _ _ _ _ _ _ w860 w875 w885 _ _ _ w909 w936 _ w958 w969 _ _ w998 w1010 w1018 _]
          tunnel: w466 -> [w476 w488 w497 w506 w510 w520 w528 w537 w542 w555 w573 w580 w592 w603 w612 w620 w632 w646 w655 w666 w675 w689 w704 w723 w737 w745 w753 w762 w770 w781 w791 w800 w811 w819 w826 w836 w861 w872 w884 w892 w898 w905 w921 w934 w948 w956 w970 w986 w993 w1000 w1012 w1020 w1022]
          tunnel: [w476 w488 w496 w505 w510 w520 w528 w536 w542 w555 w573 w580 w592 w603 w611 w620 w632 w646 w655 w666 w675 w689 w704 w723 w737 w745 w753 w762 w770 w781 w791 w800 w811 w819 w826 w836 w852 w872 w884 w892 w898 w905 w921 w934 w948 w956 w970 w986 w993 w1000 w1012 w1020 w1022] -> w465
          tunnel: [w472 w478 w491 w501 w511 w516 errorcluster {"status"=FALSE, "code"=0, "source"=""} ("error in") w531 w545 w558 w572 w578 w590 w601 w606 w622 w634 w648 w657 w668 w677 w686 w701 w717 w734 w744 w752 w761 w769 w780 w790 w794 w808 w816 w822 w829 w858 w873 w878 w888 w896 w902 w917 w924 w950 w955 w964 w985 errorcluster {"status"=FALSE, "code"=0, "source"=""} ("error in") errorcluster {"status"=FALSE, "code"=0, "source"=""} ("error in") errorcluster {"status"=FALSE, "code"=0, "source"=""} ("error in") w1015 errorcluster {"status"=FALSE, "code"=0, "source"=""} ("error out")] -> w464
          tunnel: w463 -> [_ _ _ _ _ _ _ _ _ _ w572 w578 w590 w601 _ _ _ _ _ _ _ w687 w702 _ _ w743 w751 w760 w768 w779 w789 _ w806 w814 _ w830 _ _ w878 w888 _ _ _ _ w950 _ _ w985 _ _ _ w1016 _]
          tunnel: w462 -> [_ w486 w495 w499 _ _ w523 w535 w549 w561 w568 _ w586 w598 w610 w625 w637 w651 w660 w671 w680 _ _ w726 w731 _ _ w758 w766 w777 _ w803 _ _ _ w834 w857 w871 w882 w889 w897 w904 w920 _ _ w954 _ _ _ _ _ w1019 w1025]
          tunnel: [w475 "DONE" ("value") w490 w502 w508 w519 w527 w530 w544 w557 w570 w576 w588 w599 w605 w621 w633 w647 w656 w667 w676 w690 w705 w716 w733 w739 w748 w754 w763 w771 w786 w793 w807 w815 w821 w831 w854 w863 w883 w890 w894 w900 w916 w926 w946 w952 w963 w981 w988 w999 w1011 w1017 w1023] -> w457
          tunnel: "DONE" ("response out") -> [_ _ w490 w502 w508 w519 w527 w530 w544 w557 w570 w576 w588 w599 w605 w621 w633 w647 w656 w667 w676 w690 w705 _ _ _ _ _ _ _ _ _ _ _ _ _ w854 w863 w883 w890 w894 w900 _ _ _ w952 w963 _ _ _ _ _ _]
          tunnel: w455 -> [w473 _ _ _ _ _ _ _ _ _ _ _ _ _ _ _ _ _ _ _ _ _ _ _ _ _ _ _ _ _ _ _ _ _ _ _ _ _ _ _ _ _ _ _ _ _ _ _ _ _ _ _ _]
          tunnel: "utshut" ("name") -> [_ _ _ _ _ _ _ _ _ _ _ _ _ _ _ _ _ _ _ _ _ _ _ _ _ _ _ _ _ _ _ _ _ _ _ _ _ _ w877 w887 _ _ _ _ _ _ _ _ _ _ _ _ _]
          tunnel: w453 -> [_ _ _ _ _ _ _ _ _ _ _ _ _ _ _ _ _ _ _ _ _ _ _ _ _ _ _ _ _ _ _ _ _ _ _ _ _ _ _ _ _ _ _ _ _ _ _ _ _ _ _ _ _]
          tunnel: w452 -> [_ _ _ _ _ _ _ _ _ _ _ _ _ _ _ _ _ _ _ _ _ _ _ _ _ _ _ _ _ _ _ _ _ _ _ _ _ _ _ _ _ _ _ _ _ _ _ _ w992 w999 w1011 _ _]
          tunnel: [w471 w487 0 ("return value") 0 ("return value") 0 ("return value") w514 0 ("return value") 0 ("return value") 0 ("return value") 0 ("return value") 0 ("return value") 0 ("return value") 0 ("return value") 0 ("return value") 0 ("return value") w617 0 ("return value") 0 ("return value") 0 ("return value") 0 ("return value") w672 w685 w700 0 ("return value") 0 ("return value") 0 ("return value") 0 ("return value") 0 ("return value") 0 ("return value") 0 ("return value") 0 ("return value") 0 ("return value") 0 ("return value") 0 ("return value") 0 ("return value") 0 ("return value") 0 ("return value") 0 ("return value") 0 ("return value") 0 ("return value") 0 ("return value") 0 ("return value") 0 ("return value") w925 0 ("return value") w951 w962 0 ("return value") 0 ("return value") 0 ("return value") 0 ("return value") 0 ("return value") 0 ("return value")] -> w451
          tunnel: w450 -> [_ w483 _ _ _ _ _ _ _ _ _ _ _ _ _ _ _ _ _ _ _ _ _ _ _ _ _ _ _ _ _ _ _ _ _ _ _ _ _ _ _ _ _ _ _ _ _ _ _ _ _ _ _]
          frame Default {
            n171 = call <vilib>:"Trim Whitespace.vi"("string"=w473) -> ("trimmed string"=w474:string)  [unwired: 1 in]
            n172 = call "GFITS_SetHdrVar.vi"("args"=w474) -> ("error out"=w472:errorcluster, "response"=w475:string)  [unwired: 2 in, 7 out]
            n173 = Unbundle By Name(w472) -> ("code"=w471:i32)
          }
          frame "force_headers" {
            w478 = errorcluster {"status"=FALSE, "code"=0, "source"=""} ("error out")
            n174 = call "GFITS_GetImageParams.vi"("defexts"=w483, "Database RefNum"=w486) -> ("imageStruct"=w481:T3, "CurrentReadMode"=w484:string, "header template"=w485:path)  [unwired: 7 out]
            n175 = property on="def_head_tim" class="Str"() -> ("Value"=w482:string)  [unwired: 2 in, 2 out]
            n176 = Unbundle By Name(w481) -> ("num_of_ext"=w480:u8, "multiple extensions"=w479:bool)
            n177 = call "GFITS_FillHdrGbl.vi"("mext"=w479, "ReadMode"=w484, "number of Extensions"=w480, "def_timing"=w482, "hdrfile"=w485) -> ()  [unwired: 7 out]
            n178 = Unbundle By Name(w478) -> ("code"=w487:i32)
          }
          frame "bpp" {
            n179 = Decimal String To Number(string=w498) -> (number=w492:i32)  [unwired: 3 out]
            n180 = Bundle By Name(cluster=w497, "bitpix"=w492) -> (w496:T3)
            n181 = call-poly "DatabaseHand_Set.vi"("group"="improc", "name"="bpp", "value"=w492, "Database RefNum in"=w495) -> ("error out"=w491:errorcluster)  [unwired: 4 in, 3 out]
          }
          frame "imname" {
            n182 = call "CMN_TrimStringWhitespace.vi"("string"=w504) -> ("trimmed string"=w503:string)  [unwired: 1 in, 8 out]
            n183 = Bundle By Name(cluster=w506, "name"=w503) -> (w505:T3)
            n184 = call "GFITS_SetImname.vi"("name"=w503, "Database RefNum"=w499) -> ("error out"=w501:errorcluster)  [unwired: 1 in, 8 out]
          }
          frame "imretries" {
            n185 = Scan From String(format string="%d", input string=w513) -> (error out=w511:errorcluster, output 1=→"imretries":i32)  [unwired: 2 in, 3 out]
          }
          frame "set_mbufs" {
            n186 = Scan From String(format string="%d", input string=w522) -> (error out=w517:errorcluster, output 1=w518:i32)  [unwired: 2 in, 3 out]
            n187 = To Word Integer(number=w518) -> (16bit integer=w515:i16)
            n188 = call "GFITS_LibSetNmemBufs.vi"("error in (no error)"=w517, "numbufs"=w515) -> ("error out"=w516:errorcluster, "return value"=w514:i32)  [unwired: 8 out]
          }
          frame "set_compress" {
            n189 = call "GFITS_SetCompression.vi"("cmd in"=w524, "Database RefNum out"=w523) -> ()  [unwired: 10 out]
          }
          frame "autowrit", "writetodisk" {
            n190 = call "CMN_TrimStringWhitespace.vi"("string"=w540) -> ("trimmed string"=w539:string)  [unwired: 1 in, 8 out]
            n191 = Match True/False String(2:"no" ("false string"), 3:"yes" ("true string"), 4:w539) -> (0:w533:bool)  [unwired: 1 out]
            n192 = Bundle By Name(cluster=w537, "writeToDisk"=w533) -> (w536:T3)
            n193 = call-poly "DatabaseHand_Set.vi"("group"="obs", "name"="autowrit", "value"=w533, "Database RefNum in"=w535) -> ("error out"=w531:errorcluster)  [unwired: 4 in, 3 out]
          }
          frame "fitsoverride" {
            n194 = call "CMN_TrimStringWhitespace.vi"("string"=w552) -> ("trimmed string"=w551:string)  [unwired: 1 in, 8 out]
            n195 = Match True/False String(2:"no" ("false string"), 3:"yes" ("true string"), 4:w551) -> (0:w547:bool)  [unwired: 1 out]
            n196 = call-poly "DatabaseHand_Set.vi"("group"="improc", "name"="fitsoverride", "value"=w547, "Database RefNum in"=w549) -> ("error out"=w545:errorcluster)  [unwired: 4 in, 3 out]
          }
          frame "fitsnumbering" {
            n197 = call "CMN_TrimStringWhitespace.vi"("string"=w564) -> ("trimmed string"=w563:string)  [unwired: 1 in, 8 out]
            n198 = Match True/False String(2:"no" ("false string"), 3:"yes" ("true string"), 4:w563) -> (0:w560:bool)  [unwired: 1 out]
            n199 = call-poly "DatabaseHand_Set.vi"("group"="improc", "name"="fitsnumbering", "value"=w560, "Database RefNum in"=w561) -> ("error out"=w558:errorcluster)  [unwired: 4 in, 3 out]
          }
          frame "forcename" {
            n200 = call "GFITS_ComposeNextForcedImName.vi"("argument in"=w567, "Database RefNum in"=w568) -> ("next fits"=w566:string)  [unwired: 9 out]
            n201 = local write "mImpath"(w566) -> ()
            "tmpname" <- TRUE ("tmpname")
          }
          frame "forcepath" {
            n202 = call <vilib>:"Trim Whitespace.vi"("string"=w579) -> ("trimmed string"=w574:string)  [unwired: 1 in]
            n203 = local write "tmpname"(TRUE ("tmpname")) -> ()
            n204 = local write "mImpath"(w574) -> ()
          }
          frame "testdir", "tmpdir" {
            n205 = call <vilib>:"Trim Whitespace.vi"("string"=w591) -> ("trimmed string"=w587:string)  [unwired: 1 in]
            n206 = String To Path(string=w587) -> (path=w582:path)
            n207 = call-poly "DatabaseHand_Get.vi"("default value"="test", "name"="testbname", "Database RefNum in"=w586) -> ("value"=w581:string, "Database RefNum out"=w583:T5)  [unwired: 2 in, 5 out]
            n208 = local write "testdir"(w582) -> ()
            n209 = call "GFITS_SetTestVars.vi"("testbname"=w581, "testdir"=w582, "Database RefNum in"=w583) -> ()  [unwired: 9 out]
          }
          frame "testbname" {
            n210 = call <vilib>:"Trim Whitespace.vi"("string"=w602) -> ("trimmed string"=w593:string)  [unwired: 1 in]
            n211 = local read "testdir"() -> (w595:path)
            n212 = call-poly "DatabaseHand_Get.vi"("default value"=w595, "name"="testdir", "Database RefNum in"=w598) -> ("value"=w594:path, "Database RefNum out"=w596:T5)  [unwired: 2 in, 5 out]
            n213 = call "GFITS_SetTestVars.vi"("testbname"=w593, "testdir"=w594, "Database RefNum in"=w596) -> ()  [unwired: 9 out]
          }
          frame "mext" {
            n214 = call "CMN_TrimStringWhitespace.vi"("string"=w615) -> ("trimmed string"=w614:string)  [unwired: 1 in, 8 out]
            n215 = Match True/False String(2:"no" ("false string"), 3:"yes" ("true string"), 4:w614) -> (0:w607:bool)  [unwired: 1 out]
            n216 = Bundle By Name(cluster=w612, "multiple extensions"=w607) -> (w611:T3)
            n217 = call-poly "DatabaseHand_Set.vi"("group"="image", "name"="mext", "value"=w607, "Database RefNum in"=w610) -> ("error out"=w606:errorcluster)  [unwired: 4 in, 3 out]
          }
          frame "set_memfits" {
            n218 = call "CMN_TrimStringWhitespace.vi"("string"=w628) -> ("trimmed string"=w627:string)  [unwired: 1 in, 8 out]
            n219 = Match True/False String(2:"no" ("false string"), 3:"yes" ("true string"), 4:w627) -> (0:w618:bool)  [unwired: 1 out]
            n220 = call "GFITS_LibSetMemFits.vi"("memfits"=w618) -> ("error out"=w619:errorcluster, "return value"=w617:i32)  [unwired: 1 in, 8 out]
            n221 = call-poly "DatabaseHand_Set.vi"("group"="image", "name"="memfits", "error in (no error)"=w619, "value"=w618, "Database RefNum in"=w625) -> ("error out"=w622:errorcluster)  [unwired: 3 in, 3 out]
          }
          frame "set_memhdrs" {
            n222 = call "CMN_TrimStringWhitespace.vi"("string"=w640) -> ("trimmed string"=w639:string)  [unwired: 1 in, 8 out]
            n223 = Match True/False String(2:"no" ("false string"), 3:"yes" ("true string"), 4:w639) -> (0:w631:bool)  [unwired: 1 out]
            n224 = call-poly "DatabaseHand_Set.vi"("group"="image", "name"="memhdrs", "value"=w631, "Database RefNum in"=w637) -> ("error out"=w634:errorcluster)  [unwired: 4 in, 3 out]
          }
          frame "set_postproc" {
            n225 = call "CMN_TrimStringWhitespace.vi"("string"=w645) -> ("trimmed string"=w643:string)  [unwired: 1 in, 8 out]
            n226 = call "GFITS_ParsePostProc.vi"("postproc in"=w643) -> ("postproc out"=w642:string)  [unwired: 10 out]
            n227 = property on="postproc" class="Str"("Value"=w642) -> ()  [unwired: 2 in, 2 out]
            n228 = call-poly "DatabaseHand_Set.vi"("group"="image", "name"="postproc", "value"=w642, "Database RefNum in"=w651) -> ("error out"=w648:errorcluster)  [unwired: 4 in, 3 out]
          }
          frame "set_preimg" {
            n229 = call "CMN_TrimStringWhitespace.vi"("string"=w661) -> ("trimmed string"=w653:string)  [unwired: 1 in, 8 out]
            n230 = call "GFITS_ParsePostProc.vi"("postproc in"=w653) -> ("postproc out"=w652:string)  [unwired: 10 out]
            n231 = property on="preimg" class="Str"("Value"=w652) -> ()  [unwired: 2 in, 2 out]
            n232 = call-poly "DatabaseHand_Set.vi"("group"="image", "name"="preimg", "value"=w652, "Database RefNum in"=w660) -> ("error out"=w657:errorcluster)  [unwired: 4 in, 3 out]
          }
          frame "set_postimg" {
            n233 = call "GFITS_ParsePostProc.vi"("postproc in"=w664) -> ("postproc out"=w663:string)  [unwired: 10 out]
            n234 = call "GFITS_VAR_postImgScript.vi"("script name in"=w663, "action"=enum16{"read", "write"}."write") -> ()  [unwired: 14 out]
            n235 = call-poly "DatabaseHand_Set.vi"("group"="image", "name"="postimg", "value"=w663, "Database RefNum in"=w671) -> ("error out"=w668:errorcluster)  [unwired: 4 in, 3 out]
          }
          frame "set_shmem" {
            n236 = call "CMN_TrimStringWhitespace.vi"("string"=w683) -> ("trimmed string"=w682:string)  [unwired: 1 in, 8 out]
            n237 = Match True/False String(2:"no" ("false string"), 3:"yes" ("true string"), 4:w682) -> (0:w673:bool)  [unwired: 1 out]
            n238 = call "GFITS_LibSetShmem.vi"("shmem"=w673) -> ("error out"=w674:errorcluster, "return value"=w672:i32)  [unwired: 1 in, 8 out]
            n239 = call-poly "DatabaseHand_Set.vi"("group"="image", "name"="shmem", "error in (no error)"=w674, "value"=w673, "Database RefNum in"=w680) -> ("error out"=w677:errorcluster)  [unwired: 3 in, 3 out]
          }
          frame "set_async" {
            n240 = call "CMN_TrimStringWhitespace.vi"("string"=w691) -> ("trimmed string"=w688:string)  [unwired: 1 in, 8 out]
            n241 = case shown="\"false\", \"no\", \"off\"" w688 {
              tunnel: w687 -> [_ w695 w698]
              tunnel: [errorcluster {"status"=TRUE, "code"=-22, "source"="ERROR <on | off>"} ("error out") w695 w698] -> w686
              tunnel: [-22 ("return value") 0 ("return value") 0 ("return value")] -> w685
              frame Default {
              }
              frame "on", "true", "yes" {
                n242 = property on="asyncs" class="Bool (strict)"("Value"=TRUE ("asyncs")) -> ()  [unwired: 2 in, 2 out]
              }
              frame "false", "no", "off" {
                n243 = property on="asyncs" class="Bool (strict)"("Value"=FALSE ("asyncs")) -> ()  [unwired: 2 in, 2 out]
              }
            }
          }
          frame "set_writeheaders" {
            n244 = call "CMN_TrimStringWhitespace.vi"("string"=w706) -> ("trimmed string"=w703:string)  [unwired: 1 in, 8 out]
            n245 = case shown="\"false\", \"no\", \"off\"" w703 {
              tunnel: w702 -> [_ w711 w714]
              tunnel: [errorcluster {"status"=TRUE, "code"=-22, "source"="ERROR <on | off>"} ("error out") w711 w714] -> w701
              tunnel: [-22 ("return value") 0 ("return value") 0 ("return value")] -> w700
              frame Default {
              }
              frame "on", "true", "yes" {
                n246 = property on="headers" class="Bool (strict)"("Value"=TRUE ("asyncs")) -> ()  [unwired: 2 in, 2 out]
              }
              frame "false", "no", "off" {
                n247 = property on="headers" class="Bool (strict)"("Value"=FALSE ("asyncs")) -> ()  [unwired: 2 in, 2 out]
              }
            }
          }
          frame "get_memfits" {
            n248 = call "GFITS_LibGetMemFits.vi"() -> ("error out"=w722:errorcluster, "memfits"=w721:bool)  [unwired: 1 in, 9 out]
            n249 = Append True/False String(1:w721, 2:"no" ("false string"), 3:"yes" ("true string")) -> (0:w716:string)  [unwired: 1 out]
            n250 = call-poly "DatabaseHand_Set.vi"("group"="image", "name"="memfits", "error in (no error)"=w722, "value"=w721, "Database RefNum in"=w726) -> ("error out"=w718:errorcluster)  [unwired: 3 in, 3 out]
            n251 = Bundle By Name(cluster=w718, "source"=w716) -> (w717:errorcluster)
          }
          frame "get_memhdrs" {
            n252 = call-poly "DatabaseHand_Get.vi"("default value"=FALSE, "name"="memhdrs", "Database RefNum in"=w731) -> ("error out"=w730:errorcluster, "value"=w727:bool)  [unwired: 2 in, 5 out]
            n253 = Append True/False String(1:w727, 2:"no" ("false string"), 3:"yes" ("true string")) -> (0:w733:string)  [unwired: 1 out]
            n254 = Bundle By Name(cluster=w730, "source"=w733) -> (w734:errorcluster)
          }
          frame "get_postproc" {
            n255 = property on="postproc" class="Str"() -> ("Value"=w741:string)  [unwired: 2 in, 2 out]
            n256 = Empty String/Path?(string/path=w741) -> (empty?=w742:bool)
            n257 = Select(t="none", s=w742, f=w741) -> (s? t:f=w739:string)
            n258 = Bundle By Name(cluster=w743, "source"=w739) -> (w744:errorcluster)
          }
          frame "get_preimg" {
            n259 = property on="preimg" class="Str"() -> ("Value"=w747:string)  [unwired: 2 in, 2 out]
            n260 = Empty String/Path?(string/path=w747) -> (empty?=w750:bool)
            n261 = Select(t="none", s=w750, f=w747) -> (s? t:f=w748:string)
            n262 = Bundle By Name(cluster=w751, "source"=w748) -> (w752:errorcluster)
          }
          frame "get_testdir" {
            n263 = property on="testdir" class="Path"() -> ("Value"=w755:path)  [unwired: 2 in, 2 out]
            n264 = call-poly "DatabaseHand_Get.vi"("default value"=w755, "name"="testdir", "Database RefNum in"=w758) -> ("value"=w756:path)  [unwired: 2 in, 6 out]
            n265 = Path To String(path=w756) -> (string=w754:string)
            n266 = Bundle By Name(cluster=w760, "source"=w754) -> (w761:errorcluster)
          }
          frame "get_testfname" {
            n267 = call-poly "DatabaseHand_Get.vi"("default value"="none", "name"="testfname", "Database RefNum in"=w766) -> ("value"=w763:string)  [unwired: 2 in, 6 out]
            n268 = Bundle By Name(cluster=w768, "source"=w763) -> (w769:errorcluster)
          }
          frame "get_testmode" {
            n269 = call-poly "DatabaseHand_Get.vi"("default value"=FALSE, "name"="usetestdir", "Database RefNum in"=w777) -> ("value"=w774:bool)  [unwired: 2 in, 6 out]
            n270 = Select(t="on", s=w774, f="off") -> (s? t:f=w771:string)
            n271 = Bundle By Name(cluster=w779, "source"=w771) -> (w780:errorcluster)
          }
          frame "get_postimg" {
            n272 = call "GFITS_VAR_postImgScript.vi"("action"=enum16{"read", "write"}."read") -> ("script name out"=w784:string)  [unwired: 1 in, 13 out]
            n273 = call <vilib>:"Trim Whitespace.vi"("string"=w784) -> ("trimmed string"=w782:string)  [unwired: 1 in]
            n274 = Empty String/Path?(string/path=w782) -> (empty?=w788:bool)
            n275 = Select(t="none", s=w788, f=w782) -> (s? t:f=w786:string)
            n276 = Bundle By Name(cluster=w789, "source"=w786) -> (w790:errorcluster)
          }
          frame "get_shmem" {
            n277 = call "GFITS_LibGetShmem.vi"() -> ("error out"=w799:errorcluster, "shmem"=w798:bool)  [unwired: 1 in, 9 out]
            n278 = Append True/False String(1:w798, 2:"no" ("false string"), 3:"yes" ("true string")) -> (0:w793:string)  [unwired: 1 out]
            n279 = call-poly "DatabaseHand_Set.vi"("group"="image", "name"="shmem", "error in (no error)"=w799, "value"=w798, "Database RefNum in"=w803) -> ("error out"=w795:errorcluster)  [unwired: 3 in, 3 out]
            n280 = Bundle By Name(cluster=w795, "source"=w793) -> (w794:errorcluster)
          }
          frame "get_async" {
            n281 = property on="asyncs" class="Bool (strict)"() -> ("Value"=w805:bool)  [unwired: 2 in, 2 out]
            n282 = Append True/False String(1:w805, 2:"no" ("false string"), 3:"yes" ("true string")) -> (0:w807:string)  [unwired: 1 out]
            n283 = Bundle By Name(cluster=w806, "source"=w807) -> (w808:errorcluster)
          }
          frame "get_writeheaders" {
            n284 = property on="headers" class="Bool (strict)"() -> ("Value"=w813:bool)  [unwired: 2 in, 2 out]
            n285 = Append True/False String(1:w813, 2:"no" ("false string"), 3:"yes" ("true string")) -> (0:w815:string)  [unwired: 1 out]
            n286 = Bundle By Name(cluster=w814, "source"=w815) -> (w816:errorcluster)
          }
          frame "get_membufptr" {
            n287 = call "GFITS_LibGetMemBufPtr.vi"() -> ("error out"=w823:errorcluster, "memptr"=w825:u64)  [unwired: 1 in, 9 out]
            n288 = To Unsigned Long Integer(number=w825) -> (unsigned 32bit integer=w824:u32)
            n289 = Number To Decimal String(number=w824) -> (decimal integer string=w821:string)  [unwired: 1 out]
            n290 = Bundle By Name(cluster=w823, "source"=w821) -> (w822:errorcluster)
          }
          frame "get_compress" {
            n291 = call-poly "DatabaseHand_Get.vi"("default value"="", "name"="compressfits", "Database RefNum in"=w834) -> ("value"=w833:string)  [unwired: 2 in, 6 out]
            n292 = case shown="Default" w833 {
              selector: w833 -> [w841 _]
              tunnel: [w837 "none"] -> w831
              frame Default {
                n293 = Match Pattern(string=w841, regular expression="\\[") -> (after substring=w839:string)  [unwired: 4 out]
                n294 = Match Pattern(string=w839, regular expression="\\]") -> (before substring=w837:string)  [unwired: 4 out]
              }
              frame "" {
              }
            }
            n295 = Bundle By Name(cluster=w830, "source"=w831, "status"=FALSE) -> (w829:errorcluster)
          }
          frame "num_amplifiers" {
            n296 = Scan From String(format string="%d", input string=w860) -> (error out=w858:errorcluster, output 1=w846:i32)  [unwired: 2 in, 3 out]
            n297 = Bundle By Name(cluster=w861, "num_of_ext"=w846) -> (w852:T3)
            n298 = call-poly "DatabaseHand_Set.vi"("group"="improc", "name"="num_amplifiers", "value"=w846, "Database RefNum in"=w857) -> ("error out"=w851:errorcluster, "Database RefNum out"=w850:T5)  [unwired: 4 in, 2 out]
            n299 = call-poly "DatabaseHand_Get.vi"("error in (no error)"=w851, "default value"=FALSE, "name"="mext", "Database RefNum in"=w850) -> ("value"=w847:bool)  [unwired: 1 in, 6 out]
            n300 = Select(t=w846, s=w847, f=0) -> (s? t:f=w844:i32)
            n301 = call-poly "DatabaseHand_Set.vi"("name"="num_ext", "value"=w844, "Database RefNum in"=w850) -> ()  [unwired: 5 in, 4 out]
          }
          frame "totsize" {
            w864 = "improc" ("group")
            n302 = Scan From String(format string="%d %d", input string=w875) -> (error out=w873:errorcluster, output 1=w866:i32, output 2=w865:i32)  [unwired: 2 in, 4 out]
            n303 = call-poly "DatabaseHand_Set.vi"("group"=w864, "name"="ncols", "value"=w866, "Database RefNum in"=w871) -> ("error out"=w869:errorcluster, "Database RefNum out"=w870:T5)  [unwired: 4 in, 2 out]
            n304 = call-poly "DatabaseHand_Set.vi"("group"=w864, "name"="nrows", "error in (no error)"=w869, "value"=w865, "Database RefNum in"=w870) -> ()  [unwired: 3 in, 4 out]
          }
          frame "utshut" {
            n305 = call "CMN_TrimStringWhitespace.vi"("string"=w885) -> ("trimmed string"=w880:string)  [unwired: 1 in, 8 out]
            n306 = call-poly "DatabaseHand_Set.vi"("enqueue? (F)"=TRUE, "group"="improc", "name"=w877, "value"=w880, "Database RefNum in"=w882) -> ()  [unwired: 3 in, 4 out]
          }
          frame "flushut" {
            n307 = call "DatabaseHand_FlushQvar.vi"("name"=w887, "Database RefNum In"=w889) -> ()  [unwired: 1 in, 9 out]
            n308 = call "GFITS_SeZcntProgress.vi"("counter"=0, "Database RefNum"=w889) -> ()  [unwired: 1 in, 9 out]
          }
          frame "resetprogress" {
            n309 = call "GFITS_SetWriteProgress.vi"("progress"=u8 0 ("Writeprogress"), "Database RefNum"=w897) -> ("error out"=w896:errorcluster)  [unwired: 1 in, 8 out]
          }
          frame "get_headers" {
            n310 = local read "def_head_tim"() -> (w901:string)
            n311 = call "GFITS_GetHdrTemplate.vi"("Database RefNum"=w904) -> ("path"=w903:path)  [unwired: 10 out]
            n312 = call "GFITS_GetEarlyHeaders.vi"("file"=w903, "Database RefNum in"=w904, "def_timing"=w901) -> ("error out"=w902:errorcluster)  [unwired: 1 in, 11 out]
          }
          frame "preview_headers" {
            n313 = Scan From String(format string="%s", input string=w909) -> (remaining string=w907:string, output 1=w908:string)  [unwired: 2 in, 3 out]
            n314 = Scan From String(format string="%d", input string=w907) -> (error out=w913:errorcluster, output 1=w914:i32)  [unwired: 2 in, 3 out]
            n315 = call "GFITS_GetHdrTemplate.vi"("Database RefNum"=w920) -> ("path"=w919:path)  [unwired: 10 out]
            n316 = Select(t=1, s=w913, f=w914) -> (s? t:f=w911:i32)
            n317 = call "GFITS_PreviewHeaders.vi"("file"=w919, "Database RefNum in"=w920, "extension"=w911, "timing"=w908) -> ("headers out"=w918:string[][], "error out"=w917:errorcluster)  [unwired: 2 in, 8 out]
            n318 = Flatten To String(anything=w918) -> (data string=w916:string)  [unwired: 1 in, 4 out]
          }
          frame "extensionsmap" {
            n319 = Unbundle By Name(w934) -> ("num_of_ext"=w923:u8)
            n320 = call "GFITS_Str2EXtensions.vi"("command"=w936, "curr_ext"=w923) -> ("error IO"=w935:errorcluster, "Extensions"=w932:i32[], "geom extensions"=w922:i32[])  [unwired: 1 in, 6 out]
            n321 = Array Size(array=w932) -> (size(s)=w933:i32)
            n322 = Number To Decimal String(number=w922) -> (decimal integer string=w931:string[])  [unwired: 1 out]
            n323 = call "GFITS_LibSetExtensions.vi"("error in (no error)"=w935, "num_elements"=w933, "array"=w932) -> ("error out"=w927:errorcluster)  [unwired: 8 out]
            n324 = call "CMN_Arr2Str.vi"("Array in"=w931) -> ("string out"=w929:string)  [unwired: 10 out]
            n325 = Concatenate Strings("SET EXTENSIONS " ("string"), w929) -> (w928:string)
            n326 = case shown="No Error" w927 {
              tunnel: w927 -> [w942 w945]
              tunnel: [w940 w945] -> w924
              tunnel: w928 -> [w941 _]
              tunnel: [w939 w944] -> w926
              tunnel: [w937 w943] -> w925
              frame No Error {
                n327 = call "CMN_CallGeometry.vi"("Command"=w941, "error in (no error)"=w942) -> ("ImmedReplyString"=w939:string, "error out"=w940:errorcluster)  [unwired: 12 out]
                n328 = call "CMN_testmessage.vi"("error in (no error)"=w940, "message  in"=w939) -> ("error out"=w938:errorcluster)  [unwired: 9 out]
                n329 = Unbundle By Name(w938) -> ("code"=w937:i32)
              }
              frame Error {
                n330 = Unbundle By Name(w945) -> ("source"=w944:string, "code"=w943:i32)
              }
            }
          }
          frame "get_extensionsmap" {
            n331 = Unbundle By Name(w948) -> ("num_of_ext"=w947:u8)
            n332 = call "GFITS_GetExtmap.vi"("num_ext"=w947) -> ("strout"=w946:string)  [unwired: 10 out]
          }
          frame "datacube", "nz", "zimages" {
            n333 = Scan From String(format string="%d", input string=w958) -> (output 1=w953:i32)  [unwired: 2 in, 4 out]
            n334 = call "GFITS_LibSetNzim.vi"("n z images"=w953) -> ("error out"=w955:errorcluster, "return value"=w951:i32)  [unwired: 1 in, 8 out]
            n335 = case shown="No Error" w955 {
              tunnel: w954 -> [w961 _]
              tunnel: w953 -> [w959 _]
              frame No Error {
                n336 = call-poly "DatabaseHand_Set.vi"("name"="nzim", "value"=w959, "Database RefNum in"=w961) -> ()  [unwired: 5 in, 4 out]
              }
              frame Error {
              }
            }
          }
          frame "quickhdrs" {
            n337 = Scan From String(format string="%s", input string=w969) -> (output 1=w967:string)  [unwired: 2 in, 4 out]
            n338 = To Lower Case(string=w967) -> (all lower case string=w966:string)
            n339 = case shown="\"false\", \"no\", \"off\"" w966 {
              tunnel: [w973 TRUE FALSE] -> w965
              tunnel: [errorcluster {"status"=TRUE, "code"=-22, "source"="ERROR unknown parameter"} ("error out") errorcluster {"status"=FALSE, "code"=0, "source"=""} ("error out") errorcluster {"status"=FALSE, "code"=0, "source"=""} ("error out")] -> w964
              tunnel: [-22 ("return value") 0 ("return value") 0 ("return value")] -> w962
              frame Default {
                n340 = global read "GFITS_Gbls.vi" "GFITS_quickhdrs"() -> (w973:bool)
              }
              frame "on", "true", "yes" {
              }
              frame "false", "no", "off" {
              }
            }
            n341 = global write "GFITS_Gbls.vi" "GFITS_quickhdrs"(w965) -> ()
          }
          frame "get_quickhdrs" {
            n342 = global read "GFITS_Gbls.vi" "GFITS_quickhdrs"() -> (w982:bool)
            n343 = Append True/False String(1:w982, 2:"no" ("false string"), 3:"yes" ("true string")) -> (0:w981:string)  [unwired: 1 out]
          }
          frame "get_filemsg" {
            n344 = call <vilib>:"Trim Whitespace.vi"("string"=w992) -> ("trimmed string"=w989:string)  [unwired: 1 in]
            n345 = Empty String/Path?(string/path=w989) -> (empty?=w991:bool)
            n346 = Select(t="none", s=w991, f=w989) -> (s? t:f=w988:string)
          }
          frame "set_filemsg" {
            n347 = call <vilib>:"Trim Whitespace.vi"("string"=w998) -> ("trimmed string"=w997:string)  [unwired: 1 in]
            n348 = case shown="Default" w997 {
              selector: w997 -> [w1002 _]
              tunnel: [w1002 ""] -> w996
              frame Default {
              }
              frame "disable", "none", "off" {
              }
            }
            n349 = property on="filemsg" class="Str"("Value"=w996) -> ()  [unwired: 2 in, 2 out]
          }
          frame "set_waitstats" {
            n350 = Scan From String(format string="%d", input string=w1010) -> (output 1=w1008:i32)  [unwired: 2 in, 4 out]
            n351 = Max & Min(x=w1008, y=0) -> (max(x,y)=w1006:i32)  [unwired: 1 out]
            n352 = To Unsigned Long Integer(number=w1006) -> (unsigned 32bit integer=w1005:u32)
            n353 = property on="waitstats" class="DigNum (strict)"("Value"=w1005) -> ()  [unwired: 2 in, 2 out]
          }
          frame "set_imnumformat" {
            n354 = call "GFITS_SetImNumFormat.vi"("error in"=w1016, "imnumformat"=w1018, "Database RefNum out"=w1019) -> ("error out"=w1015:errorcluster, "response"=w1017:string)  [unwired: 7 out]
          }
          frame "get_imnumformat" {
            n355 = call-poly "DatabaseHand_Get.vi"("default value"="%04d", "name"="imnumformat", "Database RefNum in"=w1025) -> ("value"=w1023:string)  [unwired: 2 in, 6 out]
          }
        }
      }
      frame "COMPUTE", "CREATE" {
        n356 = Unflatten From String(type=w1046, binary string=w1045) -> (value=w1044:T1)  [unwired: 1 in, 4 out]
        n357 = call "GFITS_GetImageParams.vi"("defexts"=w1028, "Database RefNum"=w1038) -> ("imageStruct"=w1030:T3, "header template"=w1047:path)  [unwired: 1 in, 7 out]
        n358 = Unbundle By Name(w1044) -> ("location"=w1042:u64)
        n359 = Unbundle By Name(w1030) -> ("createnewimage"=w1036:bool, "multiple extensions"=w1035:bool)
        n360 = call "GFITS_SetWriteProgress.vi"("progress"=u8 0 ("Writeprogress"), "Database RefNum"=w1038) -> ("error out"=w1032:errorcluster)  [unwired: 1 in, 8 out]
        n361 = Less Or Equal To 0?(x=w1042) -> (x <= 0?=w1043:bool)
        n362 = Select(t=w1041, s=w1043, f=w1042) -> (s? t:f=w1040:u64)
        n363 = call "GFITS_toImstats.vi"("wait"=u32 0 ("ptr"), "error in (no error)"=w1032, "cmd"="compute") -> ()  [unwired: 2 in, 7 out]
        n364 = case shown="True" w1036 {
          tunnel: [errorcluster {"status"=FALSE, "code"=0, "source"=""} ("error out") w1054] -> w1049
          tunnel: [0 ("return value") w1075] -> w1048
          tunnel: w1047 -> [_ w1071]
          tunnel: w1040 -> [w1051 w1070]
          tunnel: w1038 -> [_ w1065]
          tunnel: w1037 -> [_ w1072]
          tunnel: w1035 -> [_ w1057]
          tunnel: w1034 -> [_ w1063]
          tunnel: w1030 -> [_ w1060]
          frame False {
            n365 = property on="amplifiers" class="DigNum (strict)"("Value"=w1051) -> ()  [unwired: 2 in, 2 out]
          }
          frame True {
            n366 = call "GFITS_ExecPreImg.vi"("preimg"="preimg") -> ("error out"=w1074:errorcluster)  [unwired: 1 in, 9 out]
            n367 = property on="file reference" class="DigNum (strict)"() -> ("Value"=w1076:u64)  [unwired: 2 in, 2 out]
            n368 = call "GFITS_CloseIfValid.vi"("error in (no error)"=w1074, "fref in"=w1076) -> ("error out"=w1059:errorcluster)  [unwired: 2 in, 7 out]
            n369 = property on="image size" class="DigNum (strict)"() -> ("Value"=w1066:u32)  [unwired: 2 in, 2 out]
            n370 = local read "ReadMode"() -> (w1064:string)
            n371 = local read "mImpath"() -> (w1061:string)
            n372 = local read "tmpname"() -> (w1055:bool)
            n373 = local read "imretries"() -> (w1062:i32)
            n374 = call "GFITS_ImCreate.vi"("logfile"=w1072, "hdrfile"=w1071, "amplifiers"=w1070, "imageStruct"=w1060, "error in (no error)"=w1059, "readmode"=w1064, "headers"=w1063, "imagesize(bytes)"=w1066, "Database RefNum in"=w1065, "def_head_tim"="def_head_tim", "imretries"=w1062, "m impath in"=w1061) -> ("number of keywords"=→"number of keywords":i32[], "file reference"=→"file reference":u64, "image name out"=→"image name out":string, "expID"=→"expID":string, "error out"=w1054:errorcluster)  [unwired: 1 in, 2 out]
            n375 = case shown="True" w1055 {
              tunnel: w1054 -> [_ _]
              frame False {
              }
              frame True {
                n376 = local write "tmpname"(FALSE ("tmpname")) -> ()
                n377 = local write "mImpath"("") -> ()
              }
            }
            n378 = Unbundle By Name(w1054) -> ("code"=w1075:i32)
            "multiple extensions" <- w1057
          }
        }
      }
      frame "ABORT" {
        n379 = local read "image name out"() -> (w1087:string)
        n380 = Match Pattern(string=w1087, regular expression=".fits") -> (offset past match=w1091:i32)  [unwired: 4 out]
        n381 = Greater Than 0?(x=w1091) -> (x > 0?=w1090:bool)
        n382 = Concatenate Strings(w1087, ".fits" ("string")) -> (w1085:string)
        n383 = Select(t=w1087, s=w1090, f=w1085) -> (s? t:f=w1088:string)
        n384 = String To Path(string=w1088) -> (path=w1080:path)
        n385 = Strip Path(path=w1080) -> (stripped path=w1084:path, name=w1097:string)
        n386 = Concatenate Strings(w1097, "_ABORTED" ("string")) -> (w1095:string)
        n387 = Build Path(base path=w1084, name or relative path=w1095) -> (appended path=w1083:path)
        n388 = File/Directory Info(path=w1083) -> (path out=w1081:path, error out=w1082:errorcluster)  [unwired: 1 in, 5 out]
        n389 = case shown="Error" w1082 {
          tunnel: w1081 -> [w1101 w1102]
          tunnel: [w1100 w1102] -> w1079
          frame No Error {
            n390 = Delete(path (use dialog)=w1101) -> (deleted path=w1100:path)  [unwired: 1 in, 5 out]
          }
          frame Error {
          }
        }
        n391 = Move(source path=w1080, 10:w1079) -> ()  [unwired: 1 in, 5 out]
      }
      frame "ACQERROR" {
        n392 = flat-sequence {
          tunnel: [w1111] -> w1103
          tunnel: w1105 -> [w1119]
          tunnel: w1104 -> [w1116]
          tunnel: w1103 -> [_]
          frame #0 {
            n393 = property on="file reference" class="DigNum (strict)"() -> ("Value"=w1112:u64)  [unwired: 2 in, 2 out]
            n394 = call "GFITS_CloseIfValid.vi"("fref in"=w1112) -> ("error out"=w1111:errorcluster)  [unwired: 3 in, 7 out]
          }
          frame #1 {
            n395 = property on="expID" class="Str"() -> ("Value"=w1114:string)  [unwired: 2 in, 2 out]
            n396 = call "GFITS_GetImname.vi"("Database RefNum"=w1116) -> ("name"=w1117:string)  [unwired: 10 out]
            n397 = call "GFITS_WriteFileMsg.vi"("status"="ERROR", "expID"=w1114, "error in"=errorcluster {"status"=TRUE, "code"=0, "source"=""}, "image name (no ext)"=w1117, "filemsg"=w1119, "Database RefNum"=w1116) -> ()  [unwired: 6 out]
            n398 = property on="file reference" class="DigNum (strict)"("Value"=u64 0 ("file reference")) -> ()  [unwired: 2 in, 2 out]
          }
        }
      }
      frame "GET" {
        n399 = Scan From String(format string="%s ", input string=w1126) -> (output 1=w1127:string)  [unwired: 2 in, 4 out]
        n400 = To Upper Case(1:w1127) -> (0:w1125:string)
        n401 = case shown="\"TESTDIR\"" w1125 {
          tunnel: w1124 -> [w1134 w1140 w1146 w1152 w1158]
          tunnel: [w1132 w1138 w1144 w1150 w1156] -> w1123
          tunnel: [w1131 w1135 w1141 w1149 w1155] -> w1122
          tunnel: [w1130 w1136 w1142 w1148 w1154] -> w1121
          frame Default {
            w1130 = "ERROR unknown parameter" ("source")
            w1132 = 0 ("code")
            n402 = Bundle By Name(cluster=w1134, "status"=FALSE, "code"=w1132, "source"=w1130) -> (w1131:errorcluster)
          }
          frame "LOGFILE" {
            w1138 = 0 ("code")
            n403 = property on="logfile" class="Path"() -> ("Value"=w1137:path)  [unwired: 2 in, 2 out]
            n404 = Format Into String(w1137) -> (resulting string=w1136:string)  [unwired: 3 in, 1 out]
            n405 = Bundle By Name(cluster=w1140, "status"=FALSE, "code"=w1138, "source"=w1136) -> (w1135:errorcluster)
          }
          frame "LOGGING" {
            w1144 = 0 ("code")
            n406 = property on="log" class="Bool (strict)"() -> ("Value"=w1143:bool)  [unwired: 2 in, 2 out]
            n407 = Format Into String(w1143) -> (resulting string=w1142:string)  [unwired: 3 in, 1 out]
            n408 = Bundle By Name(cluster=w1146, "status"=FALSE, "code"=w1144, "source"=w1142) -> (w1141:errorcluster)
          }
          frame "CONFIGFILE" {
            w1150 = 0 ("code")
            n409 = property on="ConfigFile" class="Path"() -> ("Value"=w1147:path)  [unwired: 2 in, 2 out]
            n410 = Format Into String(w1147) -> (resulting string=w1148:string)  [unwired: 3 in, 1 out]
            n411 = Bundle By Name(cluster=w1152, "status"=FALSE, "code"=w1150, "source"=w1148) -> (w1149:errorcluster)
          }
          frame "TESTDIR" {
            w1156 = 0 ("code")
            n412 = property on="testdir" class="Path"() -> ("Value"=w1153:path)  [unwired: 2 in, 2 out]
            n413 = Format Into String(w1153) -> (resulting string=w1154:string)  [unwired: 3 in, 1 out]
            n414 = Bundle By Name(cluster=w1158, "status"=FALSE, "code"=w1156, "source"=w1154) -> (w1155:errorcluster)
          }
        }
      }
    }
    n415 = call "GFITS_inspectErros.vi"("message"=w142, "error in (no error)"=w146, "errno str"=w137, "error code"=w144) -> ("error out"=w124:errorcluster)  [unwired: 1 in, 6 out]
    n416 = Unbundle By Name(w124) -> ("source"=w131:string)
    n417 = call "CMN_ToServerLogQ.vi"("Log"=w130, "file"=w128, "string"=w131, "type"=w134) -> ()  [unwired: 2 in, 5 out]
    n418 = call "CMN_SetImprocError.vi"("improc error"=w124, "Database RefNum in"=w136) -> ()  [unwired: 1 in, 9 out]
    n419 = call "GFITS_responseToQ.vi"("error in"=w124, "queue name"=w122) -> ()  [unwired: 10 out]
  }
  "error out" <- w26
  n420 = case shown="True" w20 {
    tunnel: w22 -> [_ w1165]
    tunnel: w21 -> [_ w1164]
    tunnel: w19 -> [_ w1160]
    tunnel: w1 -> [_ w1159]
    frame False {
    }
    frame True {
      n421 = local read "cmd struct"() -> (w1163:T2)
      n422 = call "GFITS_dhs_server.vi"("cmdport 2"=w1165, "cmdport"=w1164) -> ()  [unwired: 10 out]
      n423 = Obtain Queue(name (unnamed)="GFITS_NetworkQ", element data type=w1163) -> (queue out=w1161:refnum<queue>)  [unwired: 3 in, 2 out]
      n424 = while {
        tunnel: w1161 -> [w1177]
        tunnel: w1160 -> [w1170]
        tunnel: w1159 -> [w1166]
        stop <- w1168 stop-if-true
        n425 = Dequeue Element(queue=w1177) -> (queue out=w1167:refnum<queue>, element=w1176:T2)  [unwired: 1 in, 3 out]
        n426 = Unbundle By Name(w1176) -> ("command"=w1172:string, "data"=w1171:string, "responseQ"=w1169:string)
        n427 = Scan From String(format string="%s", input string=w1172) -> (output 1=w1174:string)  [unwired: 2 in, 4 out]
        n428 = To Upper Case(1:w1174) -> (0:w1173:string)
        n429 = case shown="Default" w1173 {
          tunnel: w1172 -> [_ w1200]
          tunnel: w1171 -> [_ w1191]
          tunnel: w1170 -> [_ w1198]
          tunnel: w1169 -> [_ w1196]
          tunnel: [TRUE FALSE] -> w1168
          tunnel: w1167 -> [w1178 _]
          tunnel: w1166 -> [_ w1181]
          frame "SHUTDOWN" {
            n430 = Release Queue(queue=w1178) -> ()  [unwired: 1 in, 4 out]
          }
          frame Default {
            n431 = call <vilib>:"Trim Whitespace.vi"("string"=w1200) -> ("trimmed string"=w1192:string)  [unwired: 1 in]
            n432 = property on="image name out" class="Str"() -> ("Value"=w1193:string)  [unwired: 2 in, 2 out]
            n433 = property on="multiple extensions" class="Bool (strict)"() -> ("Value"=w1182:bool)  [unwired: 2 in, 2 out]
            n434 = property on="after expid" class="Str"() -> ("Value"=w1190:string)  [unwired: 2 in, 2 out]
            n435 = property on="file reference" class="DigNum (strict)"() -> ("Value"=w1194:u64)  [unwired: 2 in, 2 out]
            n436 = property on="filemsg" class="Str"() -> ("Value"=w1187:string)  [unwired: 2 in, 2 out]
            n437 = property on="expID" class="Str"() -> ("Value"=w1189:string)  [unwired: 2 in, 2 out]
            n438 = call "GFITS_Dhs_CmdHandling.vi"("imname"=w1193, "fref"=w1194, "filemsg"=w1187, "command"=w1192, "logfile"=w1181, "data"=w1191, "expID"=w1190, "mext"=w1182, "before expID"=w1189) -> ("setref"=w1180:bool, "nodeID"=w1188:string, "response"=w1186:string, "fref out"=w1183:u64, "impath"=→"mImpath":string, "error out"=w1184:errorcluster)  [unwired: 1 in]
            n439 = local write "nodeID"(w1188) -> ()
            n440 = call "GFITS_inspectErros.vi"("message"=w1186, "error in (no error)"=w1184, "errno str"=w1198, "error code"=0) -> ("error out"=w1197:errorcluster)  [unwired: 1 in, 6 out]
            n441 = case shown="True" w1180 {
              tunnel: w1183 -> [_ w1201]
              frame False {
              }
              frame True {
                n442 = property on="file reference" class="DigNum (strict)"("Value"=w1201) -> ()  [unwired: 2 in, 2 out]
              }
            }
            n443 = call "GFITS_responseToQ.vi"("error in"=w1197, "queue name"=w1196) -> ()  [unwired: 10 out]
          }
        }
      }
    }
  }
  n444 = stacked-sequence {
    tunnel: w25 -> [_]
    frame #0 {
      n445 = case shown="True" "saveconfig" {
        frame False {
        }
        frame True {
          n446 = local read "Initialization Variables"() -> (w1204:string[][])
          n447 = property on="ConfigFile" class="Path"() -> ("Value"=w1205:path)  [unwired: 2 in, 2 out]
          n448 = call "CMN_ConfigVals.vi"("Action"=enum16{"Read from File", "Write to File"}."Write to File", "ConfigVariables"=w1204, "configuration file path"=w1205) -> ()  [unwired: 1 in, 8 out]
        }
      }
      "stopped" <- TRUE
    }
  }
